vi "MoD Main-Optimize - HPLC Epoxidation Additives Simulation.vi"() -> ()   [LabVIEW 2015]
uses:
  <vilib>/silver_ctls/ArrayMatrixCluster/Real Matrix NI_Silver.ctl
  <vilib>/ni845x/ni845x.llb/ni845xControl.ctl
  <vilib>/addons/control/pid/pid.llb/PID Control Input Filter (DBL).vi
  <vilib>/addons/control/pid/autopid.llb/PID Online Autotuning (Relay Feedback).vi
  <vilib>/Analysis/Matrix/Numeric/Conversions/Array To Matrix - RA2.vi
  <vilib>/addons/control/pid/NI_PID_autopid.lvlib
  <vilib>/addons/control/pid/NI_PID_pid.lvlib
  <vilib>/Analysis/Matrix/NI_Matrix.lvlib
  <vilib>/MakerHub/LINX/LMH-LINX.lvlib
  <vilib>/MakerHub/LINX/Public/Peripherals/Digital/Digital Write 1 Chan.vi
panel:
  out "running?":bool=TRUE
  out "new_reactor_volume":bool[](array[boolean])
  out "new_reactor_length":bool[](array[boolean])
  out "Phase_Sensor_voltage":dbl
  out "P_tot":dbl
  out "pause for ms":bool=TRUE
  out "stop_xl_write":bool=TRUE
  out "Num_exp_till_pause":i32
  out "Syringe_pump?":bool=TRUE
  out "System Error":bool=TRUE
  out "error out":errorcluster
  out "Pump setpoint(ul/min) 6":dbl format="%#_13g"
  out "Pump setpoint(ul/min) 5":dbl format="%#_13g"
  out "Pump setpoint(ul/min) 4":dbl format="%#_13g"
  out "Pump setpoint(ul/min) 3":dbl format="%#_13g"
  out "Pump setpoint(ul/min) 2":dbl format="%#_13g"
  out "Pump setpoint(ul/min) 1":dbl format="%#_13g"
  out "Volume (ul) 5":dbl format="%#_13g"
  out "Volume (ul) 4":dbl format="%#_13g"
  out "Volume (ul) 3":dbl format="%#_13g"
  out "Volume (ul) 2":dbl format="%#_13g"
  out "Volume (ul) 1":dbl format="%#_13g"
  in  "tau 5":dbl format="%#_13g"
  out "tau 4":dbl format="%#_13g"
  out "tau 3":dbl format="%#_13g"
  out "tau 2":dbl format="%#_13g"
  out "tau 1":dbl format="%#_13g"
  out "Reactor Length":dbl format="%#_13g"
  out "Flowrate Sensor 2":dbl format="%#_13g"
  out "Flowrate Sensor 1":dbl format="%#_13g"
  out "Pressure 2":dbl format="%#_13g"
  out "Pressure 1":dbl format="%#_13g"
  out "Temperature Control 5":bool=TRUE
  out "Temperature Control 4":bool=TRUE
  out "Temperature Control 3":bool=TRUE
  out "Temperature Control 2":bool=TRUE
  out "Temperature Control 1":bool=TRUE
  out "Temperature SP 5":dbl format="%#_g'C"
  out "Temperature SP 4":dbl format="%#_g'C"
  out "Temperature SP 3":dbl format="%#_g'C"
  out "Temperature SP 2":dbl format="%#_g'C"
  out "Temperature SP 1":dbl format="%#_g'C"
  in  "Bay Temperature 5":dbl
  in  "SSR Duration 5":dbl
  in  "SSR Duration 4":dbl
  in  "SSR Duration 3":dbl
  in  "SSR Duration 2":dbl
  in  "SSR Duration 1":dbl
  in  "Total Product Amount":dbl=1.0 format="%#_gml"
  out "Setup Error":bool=TRUE
  out "Error Message":string
  out "ID CTR":i32
  in  "Tab Control":T1(tab)
  out "Reagent pic 5":picture
  in  "reagent name 5":string="TFE"
  out "Reagent Pic 4":picture
  in  "reagent name 4":string="ammoniumacetate"
  out "Reagent Pic 3":picture
  in  "reagent  name 3":string="Jacobsen Cat"
  in  "Product name":string="55662-89-0"
  in  "reagent name 1":string="Indene+IS(1M)"
  out "Reagent Pic 1":picture
  in  "Vr5":dbl format="%#_guL"
  in  "Vr4":dbl format="%#_guL"
  in  "Vr3":dbl format="%#_guL"
  in  "Vr2":dbl format="%#_guL"
  in  "Vr1":dbl format="%#_guL"
  in  "System decide help Button":bool
  in  "Reaction Scheme Confirm":bool
  in  "Synthesis Route Array":string[][](array[string])=[["Indene+IS(1M)", "1", "PhB(OH)2", "", "", ""], ["H2O2", "9.76", "-", "-", "-", "-"], ["Jacobsen Cat", "0.025", "-", "-", "-", "-"], ["ammoniumacetate", ".25", "-", "-", "-", "-"], ["TFE", "5", "-", "-", "-", "-"], ["Triflurotoluene", "5", "-", "-", "-", "-"]]
  in  "System decide help Button 2":bool
  out "Setup Confirm":bool=TRUE
  in  "BAY 1":u16(ring) items=["               Bypass", "         Heated Reactor", "    Small Heated Reator", "         Cooled Reactor", "      Packed Bed Reactor", "          Photo Reactor", "             Separator"]
  in  "BAY 5":u16(ring) items=["               Bypass", "         Heated Reactor", "    Small Heated Reactor", "         Cooled Reactor", "     Packed Bed Reactor", "         Photo Reactor", "             Separator"]
  in  "BAY 4":u16(ring) items=["                Bypass", "         Heated Reactor", "    Small Heated Reactor", "         Cooled Reactor", "     Packed Bed Reactor", "         Photo Reactor", "             Separator"]
  in  "BAY 3":u16(ring)=1 items=["               Bypass", "         Heated Reactor", "    Small Heated Reactor", "         Cooled Reactor", "     Packed Bed Reactor", "          Photo Reactor", "             Separator"]
  in  "BAY 2":u16(ring) items=["               Bypass", "         Heated Reactor", "    Small Heated Reactor", "         Cooled Reactor", "      Packed Bed Reactor", "          Photo Reactor", "             Separator"]
  out "Reagent Pic 2":picture
  out "Product Pic":picture
  in  "reagent name 2":string="H2O2"
  in  "reagent name 6":string="Triflurotoluene"
  out "Reagent Pic 6":picture
  in  "System Parameters Help Button":bool
  out "Setup Confirm 2":bool
  in  "System Parameters Confirm Button":bool
  in  "Bay Parameters":T2={"Bay 1 "={"Pump 1 Flowrate"=0.0, "optimize_temp"=FALSE, "optimize_tau"=TRUE, "Run at set flowrate"=FALSE, "Pump 2 Flowrate"=0.0, "Temperature Params"=[40.0, 100.0, 100.0], "pump params 1"=[5.0, 50.0, 325.0], "pump params 2"=[1.0, 10.0, 325.0], "Temperature"=0.0, "Run at set temperature"=FALSE}, "Bay 2 "={"Pump 3 Flowrate"=0.0, "optimize_temp"=FALSE, "optimize_tau"=TRUE, "Run at set flowrate"=FALSE, "Temperature Params"=[40.0, 100.0, 100.0], "Resisdence time params"=[1.0, 15.0, 650.0], "pump_at_ratio"=FALSE, "pump_num_ratio"=4.0, "Temperature"=0.0, "Run at set temperature"=FALSE}, "Bay 3 "={"Pump 4 Flowrate"=100.0, "optimize_temp"=FALSE, "optimize_tau"=TRUE, "Run at set flowrate"=FALSE, "Temperature Params"=[30.0, 50.0, 100.0], "Resisdence time params"=[0.5, 2.0, 0.0], "pump_at_ratio"=FALSE, "pump_num_ratio"=0.05, "Temperature "=0.0, "Run at set temperature"=FALSE}, "Bay 4 "={"Pump 5 Flowrate"=40.0, "Run at set flowrate"=FALSE, "optimize_temp"=FALSE, "optimize_tau"=TRUE, "Resisdence time params"=[0.5, 3.49, 225.0], "Temperature Params"=[40.0, 100.0, 80.0], "pump_at_ratio"=FALSE, "pump_num_ratio"=1.0, "Temperature"=0.0, "Run at set temperature"=FALSE}, "Bay 5 "={"Pump 6 Flowrate"=0.0, "Run at set flowrate"=FALSE, "optimize_temp"=FALSE, "optimize_tau"=FALSE, "Resisdence time params"=[7.62, 114.27, 0.0], "Temperature Params"=[0.0, 0.0, 0.0], "pump_at_ratio"=FALSE, "pump_num_ratio"=0.5, "Temperature"=0.0, "Run at set temperature"=FALSE}, "Excel File Name"="C:\\Users\\HPLC\\Dropbox (MIT)\\MoD Files\\Data\\Epox12182017", "hplc File Name"="C:\\Chem32\\1\\Data\\MOD", "Matlab File"="C:\\Users\\HPLC\\Dropbox (MIT)\\MoD Files\\Data\\Epox12182017", "Syringe for Pump 2?"=TRUE, "Num_conditons_per_wait"=2.0, "Continue from previous optimization?"=FALSE, "Total Number of Experiments 2"=60.0, "Hplc Wait time(min)"=0.25, "increas_decrease_hplc_peak"=FALSE, "Internal Standard?"=TRUE, "ISTD start"=1.2, "ISTD end"=1.9, "hplc_start"=0.7, "hplc_end"=1.1, "throughput_yield"=TRUE} {"Hplc Wait time(min)" format="%#_13g"; "Bay 5"."Temperature Params" format="%#_g'C"; "Bay 4"."Temperature Params" format="%#_g'C"; "Bay 3"."Temperature Params" format="%#_g'C"; "Bay 2"."Temperature Params" format="%#_g'C"; "Bay 1"."Temperature Params" format="%#_g'C"}
  out "System Confirm Not Clicked":string
  out "best_exp_num":dbl=1.0
  out "temperature_best":dbl[](array[numeric])
  out "Flowrates(ul/min)_best":dbl[](array[numeric])
  out "System Status":u16(ring)=2 caption="Sy" items=["System  Error", "System Running", "System Standby"]
  out "Current Experiment":dbl=1.0
  out "Total Number of Experiments":dbl=33.0
  out "Phase Sensor Chart":T3(graph)
  out "HPLC Analysis":bool
  out "Equlibrating Temperature":bool
  out "Flushing System":bool
  out "Calculate condition":bool
  out "Temperature 5":dbl format="%#_g'C"
  out "Temperature 4":dbl format="%#_g'C"
  out "Temperature 3":dbl format="%#_g'C"
  out "Temperature 2":dbl format="%#_g'C"
  out "Temperature 1":dbl format="%#_g'C"
  out "Flowrate Chart":T4(graph)
  out "Teperature Chart":T3(graph)
  out "Pump Setpoints Chart":T3(graph)
  out "Pressure Chart":T3(graph)
  out "Optimization_loop_index":i32
  out "curr_wait_time":dbl
  out "total_flush_time":dbl
  out "Temp SS? 5":bool=TRUE
  out "Temp SS? 4":bool=TRUE
  out "Temp SS? 3":bool=TRUE
  out "Temp SS? 2":bool=TRUE
  out "Temp SS? 1":bool=TRUE
  out "System Flushed?":bool
  out "stop_button clicked":bool
  in  "Pump Addresses":string[](array[string])=["g", "e", "i", "j", "f", "h", ""]
  out "experiment history":T5
  in  "Number of System Flushes per condtion":dbl=2.5
  in  "calculate volume 3":bool=TRUE
  in  "calculate volume 2":bool=TRUE
  in  "calculate volume 1":bool=TRUE
  in  "calculate volume 4":bool
  in  "calculate volume 5":bool
  in  "Extra system dead volume":dbl format="%#_gul"
  in  "new reactor length? 1":bool
  in  "tube_length(in)":dbl[](array[numeric])=[188.0, 188.0, 10.0, 10.0, 10.0]
  out "Pause Before Analysis":bool
  out "Chiller COMM Port":bool
  out "Arduino COMM Port 2":bool
  out "Temperature Sensor COMM Port":bool
  out "Flow Rate":bool
  out "Pressure":bool
  out "Pump COMM Port":bool
  in  "COMM Port :: Milligat Pumps":refnum<visa-resource-name>="COM10"
  in  "Arduino COMM Port":refnum<visa-resource-name>="COM3"
  in  "Sample Valve COMM::Port":refnum<visa-resource-name>="COM4"
  in  "COMM Port:: Harvard Syringe Pump":refnum<visa-resource-name>="COM5"
  in  "tube_id(in)":enum16{".01", ".02", ".03", ".04"}[](array[ring])=[enum.".03", enum.".03", enum.".03", enum.".03", enum.".03"]
  out "Total System Resisdence Time(min)":dbl
  in  "Debug_run_button":bool
  in  "new reactor length? 2":bool
  in  "new reactor length? 3":bool
  in  "new reactor length? 4":bool
  in  "new reactor length? 5":bool
  in  "IR Sensor Device":T6="USB0::0x3923::0x7514::01B3FF21::RAW"
  out "Stop":bool=TRUE
  in  "Run_Stop_cluster":T7
  # "Molecules on Demand"
  # "Synthetic Route"
  # "5"
  # "6"
  # "4"
  # "Product"
  # "1"
  # "2"
  # "3"
  # "Reagent List"
  # "Concentration(M)"
  # "Molecule"
  # "1"
  # "1"
  # "2"
  # "2"
  # "3"
  # "3"
  # "4"
  # "4"
  # "5"
  # "6"
  # "5"
  # "6"
  # "Product"
  # "Reactor Volume:"
  # "Optimization Parameters"
  # "Pause after"
  # "Experiments"
  # "Optimize for"
  # "to"
  # "of HPLC Peak from"
  # "from"
  # "to"
  # "min"
  # "min"
  # "HPLC runtime"
  # "# Iterations"
  # "Reporting"
  # "Excel Output File Name"
  # "HPLC File Path"
  # "MATLAB File Path"
  # "Temperature"
  # "Flowrate(ul/min)"
  # "Lower Bound"
  # "Upper Bound"
  # "Optimize?"
  # "-or-"
  # "Run at"
  # "times incoming flow"
  # "Setpoint"
  # "Temperature"
  # "Flowrate(ul/min)"
  # "Lower Bound"
  # "Upper Bound"
  # "Optimize?"
  # "-or-"
  # "Run at"
  # "times incoming flow"
  # "Setpoint"
  # "Temperature"
  # "Flowrate(ul/min)"
  # "Lower Bound"
  # "Upper Bound"
  # "Optimize?"
  # "-or-"
  # "Run at"
  # "times incoming flow"
  # "Setpoint"
  # "Temperature"
  # "Flowrate 3 (ul/min)"
  # "Lower Bound"
  # "Upper Bound"
  # "Optimize?"
  # "-or-"
  # "Run at"
  # "times incoming flow"
  # "Setpoint"
  # "Temperature"
  # "Flowrate 1(ul/min)"
  # "Flowrate 2(ul/min)"
  # "Lower Bound"
  # "Upper Bound"
  # "Optimize?"
  # "Setpoint"
  # "Pressure (psi)"
  # "System Status"
  # "Temperature('C)"
  # "BAY"
  # "1"
  # "2"
  # "3"
  # "4"
  # "5"
  # "Pump Flowrate Setpoint(ul/min)"
  # "Flowrate (ul/min)"
  # "Phase Sensor"
  # "Current Experiment"
  # "Temperature('C)"
  # "Flowrate(ul/min)"
  # "Exp"
  # "Current Best Condition"
  # "Time to reach steady state:"
  # "Current Wait Time:"
  # "Experimental Steps"
  # "Calculated New Conditions"
  # "Steady State"
  # "Analyzed HPLC"
  # "Equilibrated Temperature"
  # "Tube Length (cm)"
  # "Bay"
  # "Tube ID (in)"
  # "Calculate Volume"
  # "Use new tube length"
  # "1."
  # "2."
  # "3."
  # "4."
  # "5."
  # "Reactor Lengths\n*Heated Reactor - 188cm * Small Reactor - 99cm * Bypass - 10cm * Separator - *"
  # "1"
  # "2"
  # "3"
  # "4"
  # "5"
  # "6"
  # "All Experimental Data"
  # "P1"
  # "P2"
  # "P3"
  # "P4"
  # "P5"
  # "P6"
  # "T1"
  # "T2"
  # "T3"
  # "T4"
  # "T5"
  # "Obj_fun"
  # "HPLC_Data"
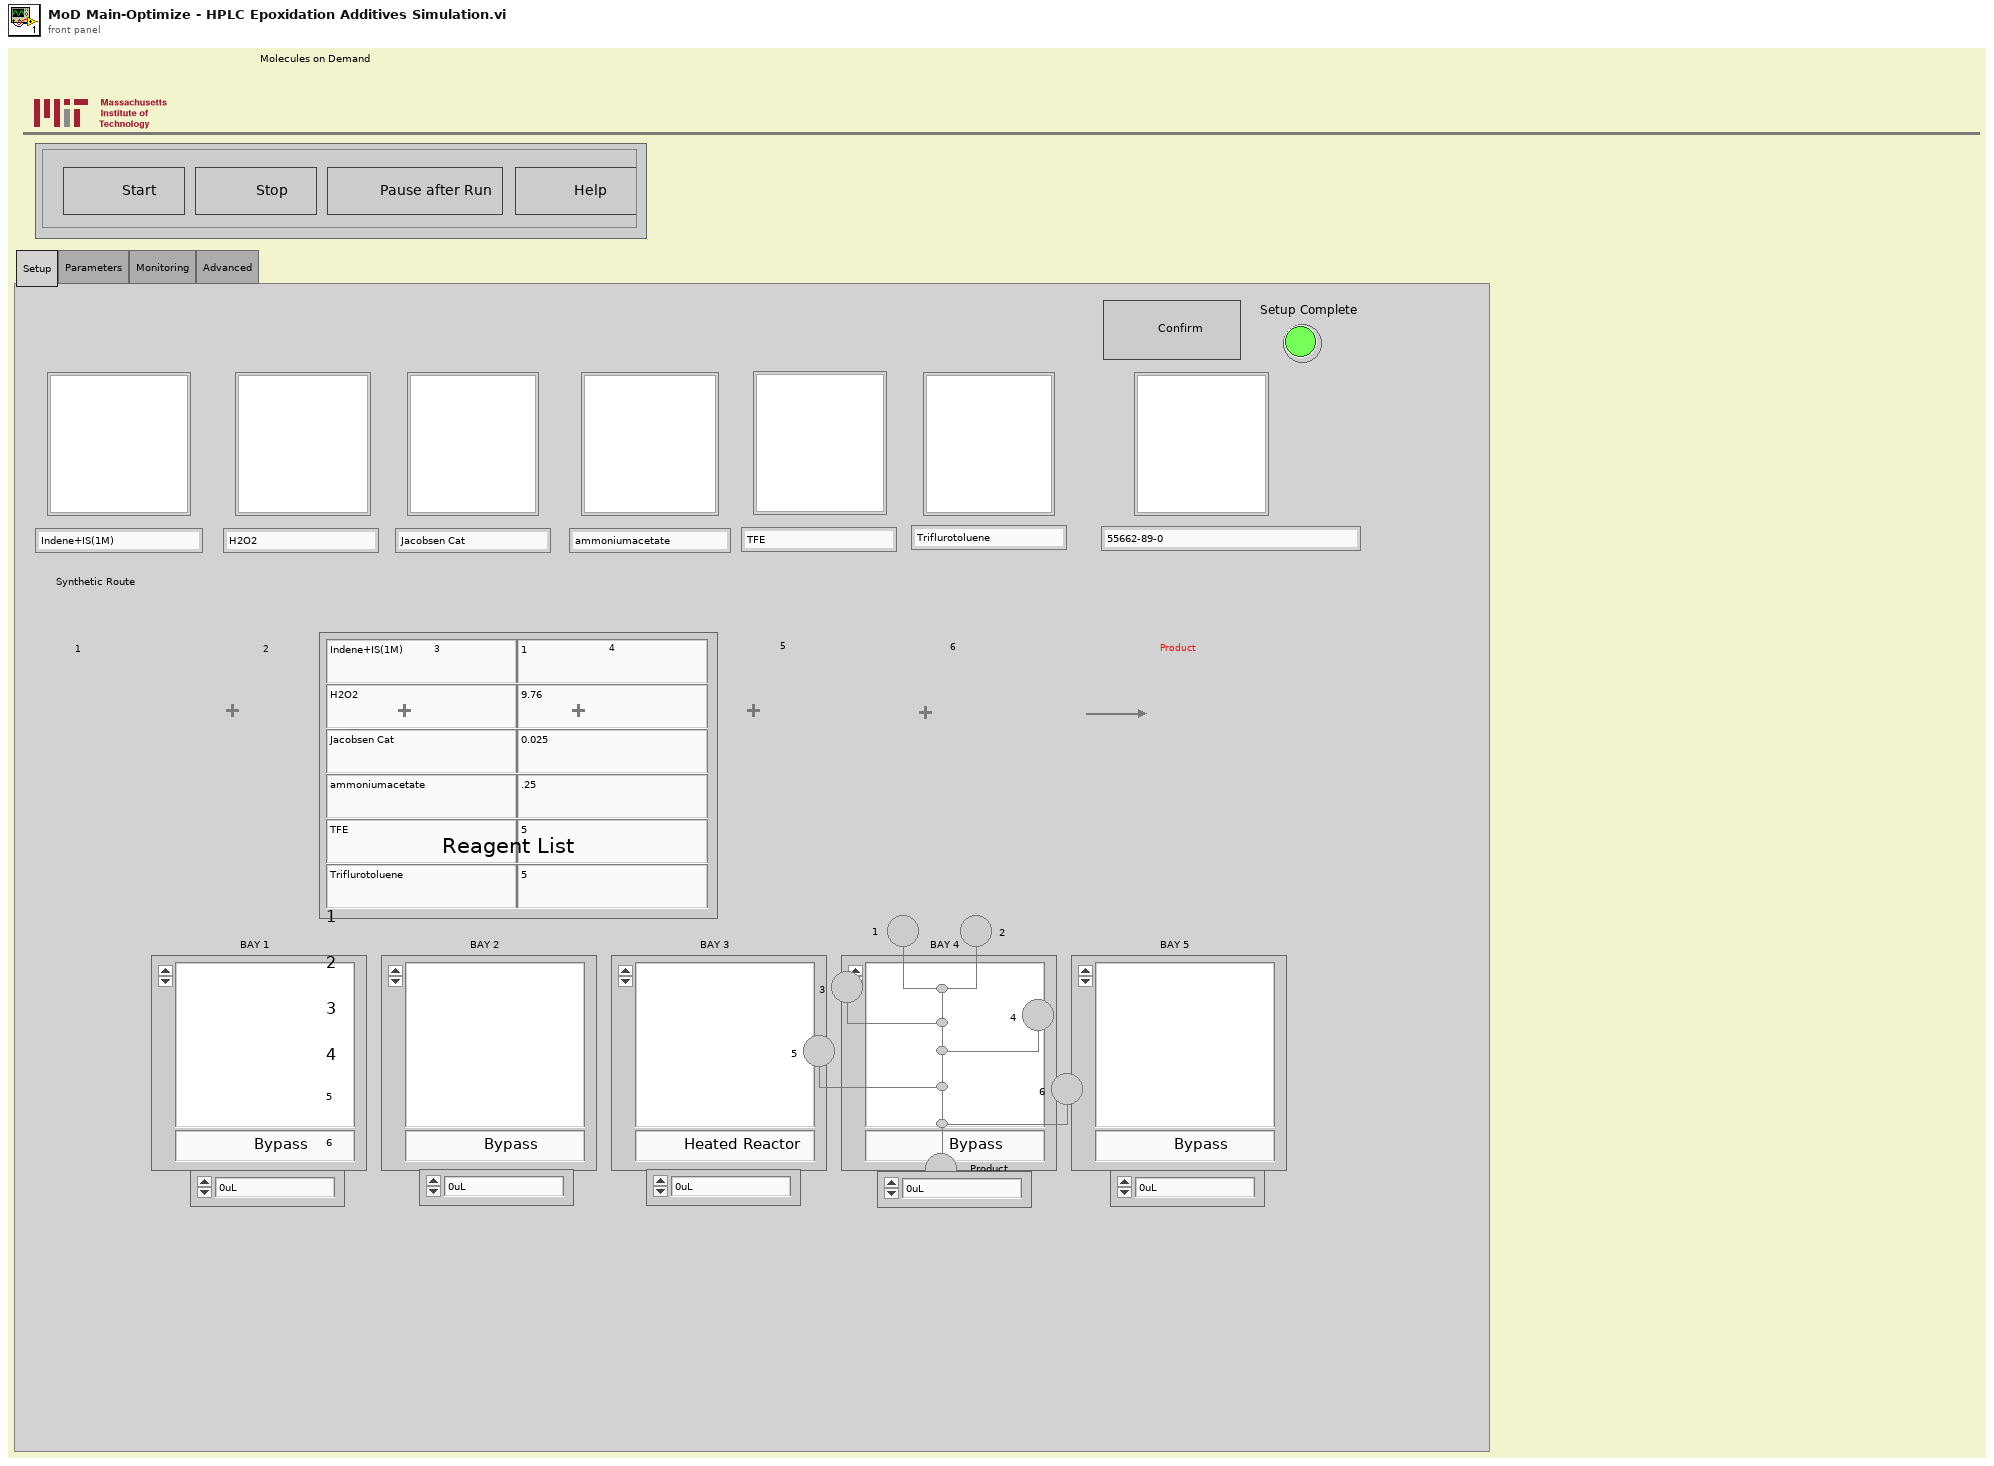
[diagram p1: front panel]
types:
  T1 = enum32{"Setup", "Parameters", "Monitoring", "Advanced"}
  T2 = cluster{"Bay 1 ":cluster{"Pump 1 Flowrate":dbl, "optimize_temp":bool, "optimize_tau":bool, "Run at set flowrate":bool, "Pump 2 Flowrate":dbl, "Temperature Params":dbl[], "pump params 1":dbl[], "pump params 2":dbl[], "Temperature":dbl, "Run at set temperature":bool}, "Bay 2 ":cluster{"Pump 3 Flowrate":dbl, "optimize_temp":bool, "optimize_tau":bool, "Run at set flowrate":bool, "Temperature Params":dbl[], "Resisdence time params":dbl[], "pump_at_ratio":bool, "pump_num_ratio":dbl, "Temperature":dbl, "Run at set temperature":bool}, "Bay 3 ":cluster{"Pump 4 Flowrate":dbl, "optimize_temp":bool, "optimize_tau":bool, "Run at set flowrate":bool, "Temperature Params":dbl[], "Resisdence time params":dbl[], "pump_at_ratio":bool, "pump_num_ratio":dbl, "Temperature ":dbl, "Run at set temperature":bool}, "Bay 4 ":cluster{"Pump 5 Flowrate":dbl, "Run at set flowrate":bool, "optimize_temp":bool, "optimize_tau":bool, "Resisdence time params":dbl[], "Temperature Params":dbl[], "pump_at_ratio":bool, "pump_num_ratio":dbl, "Temperature":dbl, "Run at set temperature":bool}, "Bay 5 ":cluster{"Pump 6 Flowrate":dbl, "Run at set flowrate":bool, "optimize_temp":bool, "optimize_tau":bool, "Resisdence time params":dbl[], "Temperature Params":dbl[], "pump_at_ratio":bool, "pump_num_ratio":dbl, "Temperature":dbl, "Run at set temperature":bool}, "Excel File Name":string, "hplc File Name":string, "Matlab File":string, "Syringe for Pump 2?":bool, "Num_conditons_per_wait":dbl, "Continue from previous optimization?":bool, "Total Number of Experiments 2":dbl, "Hplc Wait time(min)":dbl, "increas_decrease_hplc_peak":bool, "Internal Standard?":bool, "ISTD start":dbl, "ISTD end":dbl, "hplc_start":dbl, "hplc_end":dbl, "throughput_yield":bool}
  T3 = cluster{"[0]":dbl, "[1]":dbl, "[2]":dbl, "[3]":dbl, "[4]":dbl, "[5]":dbl, "[6]":dbl, "[7]":dbl, "[8]":dbl}
  T4 = cluster{"[0]":i32, "[1]":i32, "[2]":i32, "[3]":i32, "[4]":i32, "[5]":i32, "[6]":i32, "[7]":i32, "[8]":i32}
  T5 = typedef "Real Matrix NI_Silver.ctl" = dbl[][]
  T6 = typedef "ni845xControl.ctl" = refnum<k21>
  T7 = cluster{"Stop":bool, "Run":bool, "Stop Run Button":bool, "Help Button":bool}
  T8 = cluster{"Proportional gain Kc":dbl, "Integral time Ti (sec)":dbl, "Derivative time Ti (sec)":dbl}
  T9 = cluster{"type of controller":enum16{"P", "PI", "PID"}, "relay cycles":i32, "relay amplitude":dbl, "control specifications":enum16{"Fast", "Normal", "Slow"}, "PV noise level":dbl}
  T10 = typedef "imagedata.ctl" = cluster{"image type":i32, "image depth":i32, "image":u8[], "mask":u8[], "colors":u32[], "Rectangle":cluster{"left":i16, "top":i16, "right":i16, "bottom":i16}}
  T11 = cluster{"proportional gain (Kc)":dbl, "integral time (Ti, min)":dbl, "derivative time (Td, min)":dbl}
  T12 = typedef "NI_Matrix.lvlib/RealMatrix.ctl" = dbl[][]
  T13 = typedef "LMH-LINX.lvlib/LINX Ref.ctl" = cluster{"IO":T14, "Interface":T15, "LINX Device Config":T16}
  T14 = typedef "LMH-LINX.lvlib/Platform.ctl" = enum16{"Remote", "Local"}
  T15 = typedef "LMH-LINX.lvlib/Interface.ctl" = enum16{"Serial", "TCP"}
  T16 = typedef "LMH-LINX.lvlib/Device.lvlib/LINX Device Config.ctl" = cluster{"Interface":T15, "COM Port":refnum<visa-resource-name>, "TCP Configuration":T17, "Device Family":u8, "Device ID":u8, "Device Name":string, "TCP Ref":refnum<k5>, "Channels":T18}
  T17 = typedef "LMH-LINX.lvlib/Device.lvlib/TCP Config.ctl" = cluster{"IP Address":string, "Port":u16}
  T18 = typedef "LMH-LINX.lvlib/Channels.ctl" = cluster{"DI":u8[], "DO":u8[], "AI":u8[], "AO":u8[], "PWM":u8[], "QE":u8[], "UART":u8[], "I2C 2":u8[], "SPI":u8[], "CAN":u8[], "Servo":u8[], "AI Ref (V)":dbl, "AI Resolution (Bits)":u8, "AO Ref (V)":dbl, "AO Resolution (Bits)":u8}
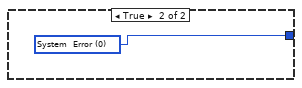
[diagram p4: hidden frame]
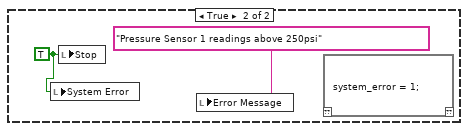
[diagram p6: hidden frame]
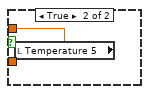
[diagram p7: hidden frame]
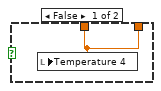
[diagram p8: hidden frame]
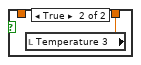
[diagram p9: hidden frame]
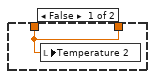
[diagram p10: hidden frame]
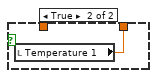
[diagram p11: hidden frame]
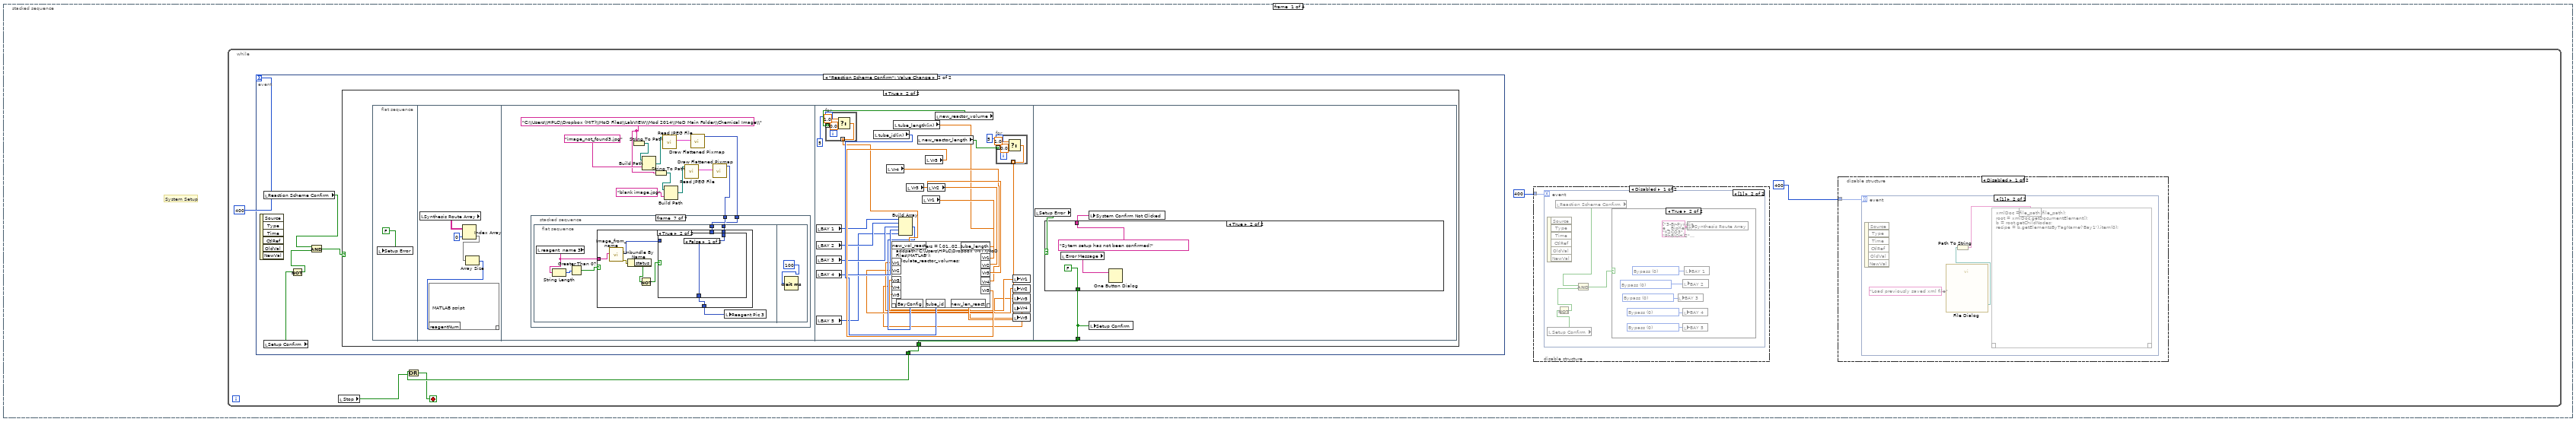
[diagram p12: hidden frame]
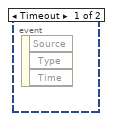
[diagram p13: hidden frame]
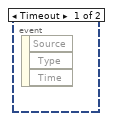
[diagram p15: hidden frame]
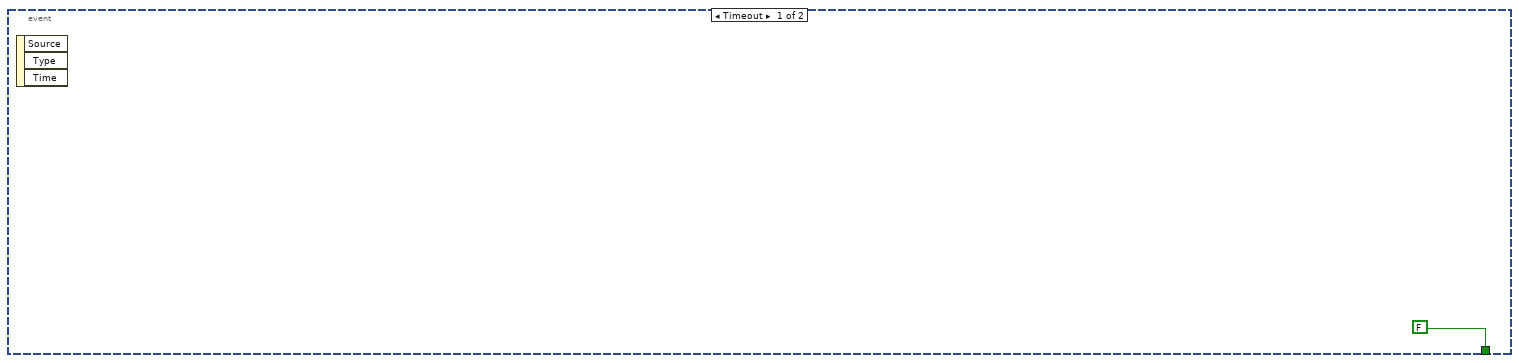
[diagram p18: hidden frame]
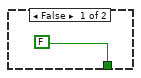
[diagram p19: hidden frame]
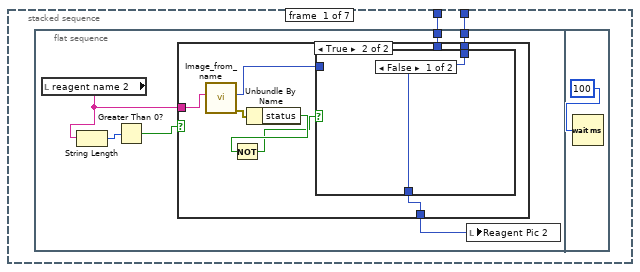
[diagram p20: hidden frame]
diagram:
  # "Assume User always uses the first bay first"
  n1 = flat-sequence {
    tunnel: ["COMM Port :: Milligat Pumps"] -> w4
    tunnel: ["Arduino COMM Port"] -> w3
    tunnel: ["Bay Parameters"] -> w1
    tunnel: [w50] -> w5
    tunnel: w4 -> [w50]
    tunnel: w3 -> [_]
    tunnel: [w44] -> w2
    tunnel: w1 -> [w41]
    tunnel: w5 -> [w54]
    tunnel: w2 -> [w53]
    frame #0 {
      w29 = FALSE ("Equlibrating Temperature")
      n2 = script code="TempArr1=[23 23 23 23 23 23 23 23 23 23]';\nTempArr2=[23 23 23 23 23 23 23 23 23 23]';\nTempArr3=[23 23 23 23 23 23 23 23 23 23]';\nTempArr4=[23 23 23 23 23 23 23 23 23 23]';\nTempArr5=[23 23 23 23 23 23 23 23 23 23]';\nTempArrLED=[23 23 23 23 23 23 23 23 23 23]';\ntemp_error1 =0;\ntemp_error2 =0;\ntemp_error3 =0;\ntemp_error4 =0;\ntemp_error5 =0;\ntemp_check1 = 0;\ntemp_check2 = 0;\ntemp_check3 = 0;\ntemp_check4 = 0;\ntemp_check5 = 0;\nT1=23;\nT2=23;\nT3=23;\nT4=23;\nT5=23;"() -> ()  [unwired: 1 in, 1 out]
      n3 = Build Array("calculate volume 1", "calculate volume 2", "calculate volume 3", "calculate volume 4", "calculate volume 5") -> (→"new_reactor_volume":bool[])
      n4 = Build Array("new reactor length? 1", "new reactor length? 2", "new reactor length? 3", "new reactor length? 4", "new reactor length? 5") -> (→"new_reactor_length":bool[])
      "Stop" <- FALSE ("Stop")
      "ID CTR" <- 0
      "Setup Confirm" <- FALSE ("Setup Confirm")
      "Error Message" <- "System shutdown sucessfully. No errors to report." ("Error Message")
      "Setup Error" <- FALSE ("Setup Error")
      "Reactor Length" <- 10.5
      "System Error" <- FALSE ("System Error")
      "Num_exp_till_pause" <- 0 ("Num_exp_till_pause")
      "Equlibrating Temperature" <- w29
      "Calculate condition" <- w29
      "Flushing System" <- w29
      "HPLC Analysis" <- w29
      "stop_xl_write" <- FALSE ("stop_xl_write")
      "Pump setpoint(ul/min) 1" <- 0.0 ("Pump setpoint(ul/min) 1")
      "Pump setpoint(ul/min) 2" <- 0.0 ("Pump setpoint(ul/min) 2")
      "Pump setpoint(ul/min) 4" <- 0.0 ("Pump setpoint(ul/min) 4")
      "Pump setpoint(ul/min) 6" <- 0.0 ("Pump setpoint(ul/min) 6")
      "Pump setpoint(ul/min) 3" <- 0.0 ("Pump setpoint(ul/min) 3")
      "Pump setpoint(ul/min) 5" <- 0.0 ("Pump setpoint(ul/min) 5")
      "pause for ms" <- FALSE ("pause for ms")
      "Setup Confirm 2" <- FALSE ("Setup Confirm 2")
      "running?" <- FALSE ("running?")
    }
    frame #1 {
      w40 = FALSE
      w49 = 23
      (unwired) path "C:/Users/User1/Documents/Lab/MoD/Images"
      n5 = disable-structure shown="Disabled" {
        frame Disabled {
          n6 = local read "BAY 2"() -> ()  [unwired: 1 out]
          n7 = local read "BAY 3"() -> ()  [unwired: 1 out]
          n8 = local read "BAY 4"() -> ()  [unwired: 1 out]
          n9 = local read "BAY 5"() -> ()  [unwired: 1 out]
          n10 = local read "BAY 1"() -> ()  [unwired: 1 out]
        }
        frame Enabled {
        }
      }
      n11 = local write "Debug_run_button"(TRUE) -> ()
      n12 = local write "System Parameters Confirm Button"(w40) -> ()
      n13 = local write "Setup Confirm 2"(w40) -> ()
      n14 = Unbundle By Name(w41) -> ("Syringe for Pump 2?"=→"Syringe_pump?":bool)
      n15 = local write "Temperature 1"(w49) -> ()
      n16 = local write "Temperature 2"(w49) -> ()
      n17 = local write "Temperature 3"(w49) -> ()
      n18 = local write "Temperature 4"(w49) -> ()
      n19 = local write "Temperature 5"(w49) -> ()
      n20 = local write "Temperature SP 1"(w49) -> ()
      n21 = local write "Temperature SP 2"(w49) -> ()
      n22 = local write "Temperature SP 3"(w49) -> ()
      n23 = local write "Temperature SP 4"(w49) -> ()
      n24 = local write "Temperature SP 5"(w49) -> ()
      n25 = Current VI's Path() -> (path=w48:path)
      n26 = Strip Path(path=w48) -> (stripped path=w46:path)  [unwired: 1 out]
      n27 = Strip Path(path=w46) -> (stripped path=w45:path)  [unwired: 1 out]
      n28 = Build Path(base path=w45, name or relative path="MATLAB") -> (appended path=w44:path)
    }
    frame #2 {
      # "Main Help Dialog Popup"
      n29 = while {
        stop <- w1206 stop-if-true
        n30 = event shown="[6] \"Run_Stop_cluster.Run\": Value Change" {
          selector: _ -> [_ _ _ _ _ _ _]
          dyn-events: _ -> [_ _ _ _ _ _ _]
          timeout: 100 -> [_ _ _ _ _ _ _]
          event Timeout {
            n31 = event-data() -> ()  [unwired: 1 in, 3 out]
          }
          event "Run_Stop_cluster.Help Button": Value Change {
            n32 = local read "Run_Stop_cluster"() -> (w1209:T7)
            n33 = event-data() -> ()  [unwired: 1 in, 4 out]
            n34 = Unbundle By Name(w1209) -> ("Help Button"=w1208:bool)
            n35 = case shown="True" w1208 {
              frame False {
              }
              frame True {
                n36 = call "help.vi"() -> ()  [unwired: 11 in]
              }
            }
          }
          event "System decide help Button": Value Change {
            n37 = event-data() -> ()  [unwired: 1 in, 5 out]
            n38 = call "help_synthesis_man-auto_instructions.vi"() -> ()  [unwired: 12 in]
          }
          event "System Parameters Help Button": Value Change {
            n39 = event-data() -> ()  [unwired: 1 in, 5 out]
            n40 = call "help_parameters_setup.vi"() -> ()  [unwired: 12 in]
          }
          event "System decide help Button 2": Value Change {
            n41 = event-data() -> ()  [unwired: 1 in, 5 out]
            n42 = call "help_synthesis_route_instructions.vi"() -> ()  [unwired: 12 in]
          }
          event "Run_Stop_cluster.Stop": Value Change {
            n43 = event-data() -> ()  [unwired: 1 in, 5 out]
            n44 = local write "Stop"(TRUE) -> ()
          }
          event "Run_Stop_cluster.Run": Value Change {
            n45 = event-data() -> ()  [unwired: 1 in, 5 out]
            n46 = local write "running?"(TRUE) -> ()
          }
        }
        n47 = local read "Stop"() -> (w1206:bool)
      }
      n48 = stacked-sequence {
        tunnel: w54 -> [_ _ _ _]
        tunnel: w53 -> [_ w392 _ _]
        frame #0 {
          # "System Setup"
          n49 = while {
            stop <- w167 stop-if-true
            n50 = event shown="[1] \"Reaction Scheme Confirm\": Value Change" {
              selector: _ -> [_ _]
              dyn-events: _ -> [_ _]
              timeout: 400 -> [_ _]
              tunnel: [FALSE w187] -> w169
              event Timeout {
                n51 = event-data() -> ()  [unwired: 1 in, 3 out]
              }
              event "Reaction Scheme Confirm": Value Change {
                n52 = event-data() -> ()  [unwired: 1 in, 6 out]
                n53 = local read "Reaction Scheme Confirm"() -> (w191:bool)
                n54 = local read "Setup Confirm"() -> (w189:bool)
                n55 = Not(x=w189) -> (.not. x?=w188:bool)
                n56 = And(x=w191, y=w188) -> (x .and. y?=w190:bool)
                n57 = case shown="True" w190 {
                  tunnel: [FALSE w193] -> w187
                  frame False {
                  }
                  frame True {
                    n58 = flat-sequence {
                      tunnel: [w382] -> w193
                      frame #0 {
                        n59 = local write "Setup Error"(FALSE) -> ()
                      }
                      frame #1 {
                        n60 = local read "Synthesis Route Array"() -> (w197:string[][])
                        n61 = Index Array(array=w197, index (col)=0 ("disabled index (col)")) -> (element=w195:string[])  [unwired: 1 in]
                        n62 = Array Size(array=w195) -> (size(s)=w198:i32)
                        n63 = script code="MATLAB script"("reagentNum"=w198) -> ()  [unwired: 1 in, 1 out]
                      }
                      frame #2 {
                        w201 = "C:\\Users\\HPLC\\Dropbox (MIT)\\MoD Files\\LabVIEW\\Mod 2014\\MoD Main Folder\\Chemical Image\\" ("string")
                        n64 = String To Path(string=w201) -> (path=w207:path)
                        n65 = Build Path(base path=w207, name or relative path="image_not_found3.jpg") -> (appended path=w206:path)
                        n66 = String To Path(string=w201) -> (path=w204:path)
                        n67 = call <vilib>:"Read JPEG File.vi"("path to JPEG file"=w206) -> ("image data"=w209:T10)  [unwired: 1 in, 9 out]
                        n68 = Build Path(base path=w204, name or relative path="blank image.jpg") -> (appended path=w202:path)
                        n69 = call <vilib>:"Read JPEG File.vi"("path to JPEG file"=w202) -> ("image data"=w205:T10)  [unwired: 1 in, 9 out]
                        n70 = call <vilib>:"Draw Flattened Pixmap.vi"("image data"=w209) -> ("new picture"=w200:picture)  [unwired: 3 in, 5 out]
                        n71 = call <vilib>:"Draw Flattened Pixmap.vi"("image data"=w205) -> ("new picture"=w199:picture)  [unwired: 3 in, 5 out]
                        n72 = stacked-sequence {
                          tunnel: w200 -> [w211 w231 w251 w271 w291 w310 w330]
                          tunnel: w199 -> [w210 w230 w250 w270 w290 w311 w331]
                          frame #0 {
                            n73 = flat-sequence {
                              tunnel: w211 -> [w217]
                              tunnel: w210 -> [w215]
                              frame #0 {
                                n74 = local read "reagent name 2"() -> (w213:string)
                                n75 = String Length(string=w213) -> (length=w216:i32)
                                n76 = Greater Than 0?(x=w216) -> (x > 0?=w214:bool)
                                n77 = case shown="True" w214 {
                                tunnel: w217 -> [_ w223]
                                tunnel: w215 -> [w218 _]
                                tunnel: [w218 w222] -> w212
                                tunnel: w213 -> [_ w221]
                                frame False {
                                }
                                frame True {
                                n78 = call "Image_from_name.vi"("Chemical Name"=w221) -> ("error out"=w224:errorcluster, "Downloaded Picture"=w225:picture)  [unwired: 8 in, 1 out]
                                n79 = Unbundle By Name(w224) -> ("status"=w220:bool)
                                n80 = Not(x=w220) -> (.not. x?=w219:bool)
                                n81 = case shown="False" w219 {
                                tunnel: w225 -> [_ w228]
                                tunnel: [w226 w227] -> w222
                                tunnel: w223 -> [w226 _]
                                frame False {
                                }
                                frame True {
                                n82 = call <vilib>:"Draw Flattened Pixmap.vi"("picture"=w228) -> ("new picture"=w227:picture)  [unwired: 8 in]
                                }
                                }
                                }
                                }
                                n83 = local write "Reagent Pic 2"(w212) -> ()
                              }
                              frame #1 {
                                n84 = Wait (ms)(milliseconds to wait=100) -> ()  [unwired: 1 out]
                              }
                            }
                          }
                          frame #1 {
                            n85 = flat-sequence {
                              tunnel: w231 -> [w237]
                              tunnel: w230 -> [w235]
                              frame #0 {
                                n86 = local read "reagent name 1"() -> (w232:string)
                                n87 = String Length(string=w232) -> (length=w236:i32)
                                n88 = Greater Than 0?(x=w236) -> (x > 0?=w234:bool)
                                n89 = case shown="True" w234 {
                                tunnel: w237 -> [_ w243]
                                tunnel: w235 -> [w238 _]
                                tunnel: [w238 w242] -> w233
                                tunnel: w232 -> [_ w241]
                                frame False {
                                }
                                frame True {
                                n90 = call "Image_from_name.vi"("Chemical Name"=w241) -> ("error out"=w244:errorcluster, "Downloaded Picture"=w245:picture)  [unwired: 8 in, 1 out]
                                n91 = Unbundle By Name(w244) -> ("status"=w240:bool)
                                n92 = Not(x=w240) -> (.not. x?=w239:bool)
                                n93 = case shown="True" w239 {
                                tunnel: w245 -> [_ w248]
                                tunnel: [w246 w247] -> w242
                                tunnel: w243 -> [w246 _]
                                frame False {
                                }
                                frame True {
                                n94 = call <vilib>:"Draw Flattened Pixmap.vi"("picture"=w248) -> ("new picture"=w247:picture)  [unwired: 8 in]
                                }
                                }
                                }
                                }
                                n95 = local write "Reagent Pic 1"(w233) -> ()
                              }
                              frame #1 {
                                n96 = Wait (ms)(milliseconds to wait=100) -> ()  [unwired: 1 out]
                              }
                            }
                          }
                          frame #2 {
                            n97 = flat-sequence {
                              tunnel: w251 -> [w257]
                              tunnel: w250 -> [w255]
                              frame #0 {
                                n98 = local read "Product name"() -> (w252:string)
                                n99 = String Length(string=w252) -> (length=w256:i32)
                                n100 = Greater Than 0?(x=w256) -> (x > 0?=w254:bool)
                                n101 = case shown="True" w254 {
                                tunnel: w257 -> [_ w263]
                                tunnel: w255 -> [w258 _]
                                tunnel: [w258 w262] -> w253
                                tunnel: w252 -> [_ w261]
                                frame False {
                                }
                                frame True {
                                n102 = call "Image_from_name.vi"("Chemical Name"=w261) -> ("error out"=w264:errorcluster, "Downloaded Picture"=w265:picture)  [unwired: 8 in, 1 out]
                                n103 = Unbundle By Name(w264) -> ("status"=w259:bool)
                                n104 = Not(x=w259) -> (.not. x?=w260:bool)
                                n105 = case shown="False" w260 {
                                tunnel: w265 -> [_ w268]
                                tunnel: [w266 w267] -> w262
                                tunnel: w263 -> [w266 _]
                                frame False {
                                }
                                frame True {
                                n106 = call <vilib>:"Draw Flattened Pixmap.vi"("picture"=w268) -> ("new picture"=w267:picture)  [unwired: 8 in]
                                }
                                }
                                }
                                }
                                n107 = local write "Product Pic"(w253) -> ()
                              }
                              frame #1 {
                                n108 = Wait (ms)(milliseconds to wait=100) -> ()  [unwired: 1 out]
                              }
                            }
                          }
                          frame #3 {
                            n109 = flat-sequence {
                              tunnel: w271 -> [w277]
                              tunnel: w270 -> [w275]
                              frame #0 {
                                n110 = local read "reagent name 6"() -> (w272:string)
                                n111 = String Length(string=w272) -> (length=w276:i32)
                                n112 = Greater Than 0?(x=w276) -> (x > 0?=w274:bool)
                                n113 = case shown="True" w274 {
                                tunnel: w277 -> [_ w283]
                                tunnel: w275 -> [w278 _]
                                tunnel: [w278 w282] -> w273
                                tunnel: w272 -> [_ w281]
                                frame False {
                                }
                                frame True {
                                n114 = call "Image_from_name.vi"("Chemical Name"=w281) -> ("error out"=w284:errorcluster, "Downloaded Picture"=w285:picture)  [unwired: 8 in, 1 out]
                                n115 = Unbundle By Name(w284) -> ("status"=w279:bool)
                                n116 = Not(x=w279) -> (.not. x?=w280:bool)
                                n117 = case shown="False" w280 {
                                tunnel: w285 -> [_ w288]
                                tunnel: [w286 w287] -> w282
                                tunnel: w283 -> [w286 _]
                                frame False {
                                }
                                frame True {
                                n118 = call <vilib>:"Draw Flattened Pixmap.vi"("picture"=w288) -> ("new picture"=w287:picture)  [unwired: 8 in]
                                }
                                }
                                }
                                }
                                n119 = local write "Reagent Pic 6"(w273) -> ()
                              }
                              frame #1 {
                                n120 = Wait (ms)(milliseconds to wait=100) -> ()  [unwired: 1 out]
                              }
                            }
                          }
                          frame #4 {
                            n121 = flat-sequence {
                              tunnel: w291 -> [w297]
                              tunnel: w290 -> [w295]
                              frame #0 {
                                n122 = local read "reagent name 5"() -> (w292:string)
                                n123 = String Length(string=w292) -> (length=w296:i32)
                                n124 = Greater Than 0?(x=w296) -> (x > 0?=w294:bool)
                                n125 = case shown="True" w294 {
                                tunnel: w297 -> [_ w303]
                                tunnel: w295 -> [w298 _]
                                tunnel: [w298 w302] -> w293
                                tunnel: w292 -> [_ w301]
                                frame False {
                                }
                                frame True {
                                n126 = call "Image_from_name.vi"("Chemical Name"=w301) -> ("error out"=w304:errorcluster, "Downloaded Picture"=w305:picture)  [unwired: 8 in, 1 out]
                                n127 = Unbundle By Name(w304) -> ("status"=w299:bool)
                                n128 = Not(x=w299) -> (.not. x?=w300:bool)
                                n129 = case shown="False" w300 {
                                tunnel: w305 -> [_ w308]
                                tunnel: [w306 w307] -> w302
                                tunnel: w303 -> [w306 _]
                                frame False {
                                }
                                frame True {
                                n130 = call <vilib>:"Draw Flattened Pixmap.vi"("picture"=w308) -> ("new picture"=w307:picture)  [unwired: 8 in]
                                }
                                }
                                }
                                }
                                n131 = local write "Reagent pic 5"(w293) -> ()
                              }
                              frame #1 {
                                n132 = Wait (ms)(milliseconds to wait=100) -> ()  [unwired: 1 out]
                              }
                            }
                          }
                          frame #5 {
                            n133 = flat-sequence {
                              tunnel: w311 -> [w315]
                              tunnel: w310 -> [w314]
                              frame #0 {
                                n134 = local read "reagent name 4"() -> (w312:string)
                                n135 = String Length(string=w312) -> (length=w317:i32)
                                n136 = Greater Than 0?(x=w317) -> (x > 0?=w316:bool)
                                n137 = case shown="True" w316 {
                                tunnel: w314 -> [_ w323]
                                tunnel: w315 -> [w318 _]
                                tunnel: [w318 w322] -> w313
                                tunnel: w312 -> [_ w321]
                                frame False {
                                }
                                frame True {
                                n138 = call "Image_from_name.vi"("Chemical Name"=w321) -> ("error out"=w324:errorcluster, "Downloaded Picture"=w325:picture)  [unwired: 8 in, 1 out]
                                n139 = Unbundle By Name(w324) -> ("status"=w319:bool)
                                n140 = Not(x=w319) -> (.not. x?=w320:bool)
                                n141 = case shown="False" w320 {
                                tunnel: w325 -> [_ w328]
                                tunnel: [w326 w327] -> w322
                                tunnel: w323 -> [w326 _]
                                frame False {
                                }
                                frame True {
                                n142 = call <vilib>:"Draw Flattened Pixmap.vi"("picture"=w328) -> ("new picture"=w327:picture)  [unwired: 8 in]
                                }
                                }
                                }
                                }
                                n143 = local write "Reagent Pic 4"(w313) -> ()
                              }
                              frame #1 {
                                n144 = Wait (ms)(milliseconds to wait=100) -> ()  [unwired: 1 out]
                              }
                            }
                          }
                          frame #6 {
                            n145 = flat-sequence {
                              tunnel: w331 -> [w335]
                              tunnel: w330 -> [w334]
                              frame #0 {
                                n146 = local read "reagent  name 3"() -> (w332:string)
                                n147 = String Length(string=w332) -> (length=w337:i32)
                                n148 = Greater Than 0?(x=w337) -> (x > 0?=w336:bool)
                                n149 = case shown="True" w336 {
                                tunnel: w334 -> [_ w343]
                                tunnel: w335 -> [w338 _]
                                tunnel: [w338 w342] -> w333
                                tunnel: w332 -> [_ w341]
                                frame False {
                                }
                                frame True {
                                n150 = call "Image_from_name.vi"("Chemical Name"=w341) -> ("error out"=w344:errorcluster, "Downloaded Picture"=w345:picture)  [unwired: 8 in, 1 out]
                                n151 = Unbundle By Name(w344) -> ("status"=w339:bool)
                                n152 = Not(x=w339) -> (.not. x?=w340:bool)
                                n153 = case shown="False" w340 {
                                tunnel: w345 -> [_ w348]
                                tunnel: [w346 w347] -> w342
                                tunnel: w343 -> [w346 _]
                                frame False {
                                }
                                frame True {
                                n154 = call <vilib>:"Draw Flattened Pixmap.vi"("picture"=w348) -> ("new picture"=w347:picture)  [unwired: 8 in]
                                }
                                }
                                }
                                }
                                n155 = local write "Reagent Pic 3"(w333) -> ()
                              }
                              frame #1 {
                                n156 = Wait (ms)(milliseconds to wait=100) -> ()  [unwired: 1 out]
                              }
                            }
                          }
                        }
                      }
                      frame #3 {
                        n157 = local read "BAY 1"() -> (w360:u16)
                        n158 = local read "BAY 2"() -> (w359:u16)
                        n159 = local read "BAY 3"() -> (w358:u16)
                        n160 = local read "BAY 4"() -> (w357:u16)
                        n161 = local read "BAY 5"() -> (w356:u16)
                        n162 = local read "tube_id(in)"() -> (w367:enum16{".01", ".02", ".03", ".04"}[])
                        n163 = local read "Vr4"() -> (w370:dbl)
                        n164 = local read "tube_length(in)"() -> (w368:dbl[])
                        n165 = Build Array(w360, w359, w358, w357, w356) -> (w355:u16[])
                        n166 = local read "Vr3"() -> (w371:dbl)
                        n167 = local read "new_reactor_length"() -> (w365:bool[])
                        n168 = local read "Vr1"() -> (w373:dbl)
                        n169 = local read "Vr5"() -> (w369:dbl)
                        n170 = local read "Vr2"() -> (w372:dbl)
                        n171 = local read "new_reactor_volume"() -> (w363:bool[])
                        n172 = for {
                          N: 5 -> [_]
                          tunnel: w363 -> [w377] mode=indexing
                          tunnel: [w374] -> w361 mode=indexing
                          n173 = Select(t=1.0, s=w377, f=0.0) -> (s? t:f=w374:dbl)
                        }
                        n174 = for {
                          N: 5 -> [_]
                          tunnel: w365 -> [w381] mode=indexing
                          tunnel: [w378] -> w364 mode=indexing
                          n175 = Select(t=1.0, s=w381, f=0.0) -> (s? t:f=w378:dbl)
                        }
                        n176 = script code="tube_diameters = [.01,.02,.03,.04];\naddpath('C:\\Users\\HPLC\\Dropbox (MIT)\\MoD Files\\MATLAB');\ncalculate_reactor_volumes;"("BayConfig"=w355, "Vr1"=w373, "Vr2"=w372, "Vr3"=w371, "Vr4"=w370, "Vr5"=w369, "tube_length"=w368, "tube_id"=w367, "new_len_react"=w364, "new_vol_react"=w361) -> ("Vr1"=w354:dbl, "Vr2"=w353:dbl, "Vr3"=w352:dbl, "Vr4"=w351:dbl, "Vr5"=w350:dbl)  [unwired: 1 in, 1 out]
                        n177 = local write "Vr1"(w354) -> ()
                        n178 = local write "Vr2"(w353) -> ()
                        n179 = local write "Vr3"(w352) -> ()
                        n180 = local write "Vr4"(w351) -> ()
                        n181 = local write "Vr5"(w350) -> ()
                      }
                      frame #4 {
                        n182 = local read "Setup Error"() -> (w384:bool)
                        n183 = case shown="True" w384 {
                          tunnel: [TRUE FALSE] -> w382
                          tunnel: ["" "Sytem setup has not been confirmed!"] -> w383
                          frame False {
                          }
                          frame True {
                            n184 = local read "Error Message"() -> (w389:string)
                            n185 = One Button Dialog(message=w389) -> ()  [unwired: 1 in, 1 out]
                          }
                        }
                        n186 = local write "System Confirm Not Clicked"(w383) -> ()
                        n187 = local write "Setup Confirm"(w382) -> ()
                      }
                    }
                  }
                }
              }
            }
            n188 = local read "Stop"() -> (w168:bool)
            n189 = Or(x=w169, y=w168) -> (x .or. y?=w167:bool)
            n190 = disable-structure shown="Disabled" {
              disable-tunnel: 400 -> [w175 _]
              frame Disabled {
                n191 = event shown="[1]" {
                  selector: _ -> [_ _]
                  dyn-events: _ -> [_ _]
                  timeout: w175 -> [_ _]
                  event Timeout {
                    n192 = event-data() -> ()  [unwired: 1 in, 3 out]
                  }
                  event #1 (no event record) {
                    n193 = event-data() -> ()  [unwired: 1 in, 6 out]
                    n194 = local read "Setup Confirm"() -> (w176:bool)
                    n195 = local read "Reaction Scheme Confirm"() -> (w177:bool)
                    n196 = Not(x=w176) -> (.not. x?=w179:bool)
                    n197 = And(x=w177, y=w179) -> (x .and. y?=w178:bool)
                    n198 = case shown="True" w178 {
                      frame False {
                      }
                      frame True {
                        w181 = u16 0 items=["                     Bypass", "                Hot Reactor", "                 Separator"] ("BAY 5")
                        w182 = u16 0 items=["                     Bypass", "                Hot Reactor", "                  Separator"] ("BAY 4")
                        w183 = u16 0 items=["                     Bypass", "                 Hot Reactor", "                  Separator"] ("BAY 3")
                        w184 = u16 0 items=["                     Bypass", "                Hot Reactor", "                  Separator"] ("BAY 2")
                        w185 = u16 0 items=["                 Bypass", "             Hot Reactor", "               Separator"] ("BAY 1")
                        n199 = local write "BAY 3"(w183) -> ()
                        n200 = local write "BAY 4"(w182) -> ()
                        n201 = local write "BAY 5"(w181) -> ()
                        n202 = local write "BAY 2"(w184) -> ()
                        n203 = local write "BAY 1"(w185) -> ()
                        n204 = local write "Synthesis Route Array"(string[][] [["3-Br-Pyridine _ Biphenyl", "K2CO3", "PhB(OH)2", "", "", ""]] ("Synthesis Route Array")) -> ()
                      }
                    }
                  }
                }
              }
              frame Enabled {
              }
            }
            n205 = disable-structure shown="Disabled" {
              disable-tunnel: 400 -> [w171 _]
              frame Disabled {
                n206 = event shown="[1]" {
                  selector: _ -> [_ _]
                  dyn-events: _ -> [_ _]
                  timeout: w171 -> [_ _]
                  event Timeout {
                    n207 = event-data() -> ()  [unwired: 1 in, 3 out]
                  }
                  event #1 (no event record) {
                    n208 = event-data() -> ()  [unwired: 1 in, 6 out]
                    n209 = call "File Dialog"("prompt"="Load previously saved xml file") -> ("selected path"=w173:path)  [unwired: 11 in, 3 out]
                    n210 = Path To String(path=w173) -> (string=w172:string)
                    n211 = script code="xmlDoc = xmlread(file_path);\nroot = xmlDoc.getDocumentElement();\nb = root.getChildNodes;\nrecipe = b.getElementsByTagName('Bay1').item(0);"("file_path"=w172) -> ()  [unwired: 1 in, 1 out]
                  }
                }
              }
              frame Enabled {
              }
            }
          }
        }
        frame #1 {
          n212 = local read "Stop"() -> (w391:bool)
          n213 = Not(x=w391) -> (.not. x?=w390:bool)
          n214 = case shown="True" w390 {
            tunnel: w392 -> [_ w395]
            frame False {
              "stop_button clicked" <- TRUE ("stop_button clicked")
            }
            frame True {
              # "Parameters Initilization"
              n215 = flat-sequence {
                tunnel: w395 -> [w397]
                tunnel: [w396] -> w394
                tunnel: w394 -> [w556]
                frame #0 {
                  # "Setup bays(RFID - verify)"
                  n216 = disable-structure shown="Disabled" {
                    frame Disabled {
                      n217 = local read "BAY 1"() -> ()  [unwired: 1 out]
                      n218 = local read "BAY 2"() -> ()  [unwired: 1 out]
                      n219 = local read "BAY 3"() -> ()  [unwired: 1 out]
                      n220 = local read "BAY 4"() -> ()  [unwired: 1 out]
                      n221 = local read "BAY 5"() -> ()  [unwired: 1 out]
                    }
                    frame Enabled {
                    }
                  }
                }
                frame #1 {
                  n222 = while {
                    tunnel: w397 -> [w400]
                    tunnel: [w399] -> w396
                    stop <- w403 stop-if-true
                    n223 = flat-sequence {
                      tunnel: [w417] -> w399
                      tunnel: w400 -> [w498]
                      tunnel: [w416] -> w398
                      frame #0 {
                        n224 = while {
                          stop <- w407 stop-if-true
                          n225 = event shown="[1] \"System Parameters Confirm Button\": Value Change" {
                            selector: _ -> [_ _]
                            dyn-events: _ -> [_ _]
                            timeout: u32 200 ("milliseconds to wait") -> [_ _]
                            tunnel: [FALSE TRUE] -> w405
                            event Timeout {
                              n226 = event-data() -> ()  [unwired: 1 in, 3 out]
                            }
                            event "System Parameters Confirm Button": Value Change {
                              n227 = event-data() -> ()  [unwired: 1 in, 5 out]
                              n228 = local write "System Parameters Confirm Button"(FALSE) -> ()
                            }
                          }
                          n229 = Wait (ms)(milliseconds to wait=u32 500) -> ()  [unwired: 1 out]
                          n230 = local read "Stop"() -> (w408:bool)
                          n231 = Or(x=w408, y=w405) -> (x .or. y?=w407:bool)
                        }
                      }
                      frame #1 {
                        w437 = 0 ("disabled index (col)")
                        w449 = 1 ("disabled index (col)")
                        # "Do while parameters have not been correctly entered"
                        n232 = local read "Bay Parameters"() -> (w436:T2)
                        n233 = local read "Synthesis Route Array"() -> (w450:string[][])
                        n234 = local read "Total Number of Experiments"() -> (w469:dbl)
                        n235 = Unbundle By Name(w436) -> ("Continue from previous optimization?"=w497:bool)
                        n236 = Unbundle By Name(w436) -> ("Excel File Name"=w499:string)
                        n237 = Unbundle By Name(w436) -> ("Matlab File"=w495:string)
                        n238 = Unbundle By Name(w436) -> ("Bay 1.Run at set flowrate"=w541:bool)
                        n239 = Unbundle By Name(w436) -> ("Bay 1.Pump 1 Flowrate"=w547:dbl)
                        n240 = Unbundle By Name(w436) -> ("Bay 1.Pump 2 Flowrate"=w546:dbl)
                        n241 = Unbundle By Name(w436) -> ("Bay 2.Run at set flowrate"=w539:bool)
                        n242 = Unbundle By Name(w436) -> ("Bay 2.Pump 3 Flowrate"=w545:dbl)
                        n243 = Unbundle By Name(w436) -> ("Bay 3.Pump 4 Flowrate"=w544:dbl)
                        n244 = Unbundle By Name(w436) -> ("Bay 3.Run at set flowrate"=w538:bool)
                        n245 = Unbundle By Name(w436) -> ("Bay 4.Run at set flowrate"=w535:bool)
                        n246 = Unbundle By Name(w436) -> ("Bay 4.Pump 5 Flowrate"=w543:dbl)
                        n247 = Unbundle By Name(w436) -> ("Bay 5.Pump 6 Flowrate"=w542:dbl)
                        n248 = Unbundle By Name(w436) -> ("Bay 5.Run at set flowrate"=w534:bool)
                        n249 = Index Array(array=w450, index (row)=3, index (col)=w449) -> (element=w443:string)
                        n250 = Index Array(array=w450, index (row)=2, index (col)=w449) -> (element=w441:string)
                        n251 = Index Array(array=w450, index (row)=1, index (col)=w449) -> (element=w439:string)
                        n252 = Index Array(array=w450, index (row)=0, index (col)=w449) -> (element=w452:string)
                        n253 = Index Array(array=w450, index (row)=4, index (col)=w449) -> (element=w445:string)
                        n254 = Index Array(array=w450, index (row)=5, index (col)=w449) -> (element=w447:string)
                        n255 = Build Array(w452, w439, w441, w443, w445, w447) -> (w453:string[])
                        n256 = Index Array(array=w450, index (row)=0 ("index"), index (col)=w437) -> (element=w475:string)
                        n257 = for {
                          tunnel: w453 -> [w549] mode=indexing
                          tunnel: [w548] -> w438 mode=indexing
                          n258 = script code="ctemp1 = str2num(c_temp);"("c_temp"=w549) -> ("ctemp1"=w548:dbl)  [unwired: 1 in, 1 out]
                        }
                        n259 = Boolean To (0,1)(Boolean=w539) -> (0, 1=w494:i16)
                        n260 = Boolean To (0,1)(Boolean=w535) -> (0, 1=w536:i16)
                        n261 = Boolean To (0,1)(Boolean=w538) -> (0, 1=w537:i16)
                        n262 = Boolean To (0,1)(Boolean=w497) -> (0, 1=w496:i16)
                        n263 = Boolean To (0,1)(Boolean=w541) -> (0, 1=w540:i16)
                        n264 = Boolean To (0,1)(Boolean=w534) -> (0, 1=w533:i16)
                        n265 = Index Array(array=w450, index (row)=1 ("index"), index (col)=w437) -> (element=w470:string)
                        n266 = Index Array(array=w450, index (row)=2 ("index"), index (col)=w437) -> (element=w471:string)
                        n267 = Unbundle By Name(w436) -> ("Bay 1.optimize_temp"=w532:bool)
                        n268 = Unbundle By Name(w436) -> ("Bay 1.optimize_tau"=w530:bool)
                        n269 = Unbundle By Name(w436) -> ("Bay 2.optimize_temp"=w528:bool)
                        n270 = Unbundle By Name(w436) -> ("Bay 2.optimize_tau"=w526:bool)
                        n271 = Unbundle By Name(w436) -> ("Bay 3.optimize_temp"=w524:bool)
                        n272 = Unbundle By Name(w436) -> ("Bay 3.optimize_tau"=w522:bool)
                        n273 = Unbundle By Name(w436) -> ("Bay 4.optimize_temp"=w520:bool)
                        n274 = Unbundle By Name(w436) -> ("Bay 4.optimize_tau"=w518:bool)
                        n275 = Index Array(array=w450, index (row)=3 ("index"), index (col)=w437) -> (element=w472:string)
                        n276 = Boolean To (0,1)(Boolean=w520) -> (0, 1=w519:i16)
                        n277 = Boolean To (0,1)(Boolean=w518) -> (0, 1=w517:i16)
                        n278 = Index Array(array=w450, index (row)=4 ("index"), index (col)=w437) -> (element=w473:string)
                        n279 = Boolean To (0,1)(Boolean=w522) -> (0, 1=w521:i16)
                        n280 = Boolean To (0,1)(Boolean=w528) -> (0, 1=w527:i16)
                        n281 = Boolean To (0,1)(Boolean=w532) -> (0, 1=w531:i16)
                        n282 = Boolean To (0,1)(Boolean=w526) -> (0, 1=w525:i16)
                        n283 = Boolean To (0,1)(Boolean=w530) -> (0, 1=w529:i16)
                        n284 = Boolean To (0,1)(Boolean=w524) -> (0, 1=w523:i16)
                        n285 = Unbundle By Name(w436) -> ("Bay 5.optimize_temp"=w516:bool)
                        n286 = Unbundle By Name(w436) -> ("Bay 5.optimize_tau"=w514:bool)
                        n287 = Index Array(array=w450, index (row)=5 ("index"), index (col)=w437) -> (element=w474:string)
                        n288 = Boolean To (0,1)(Boolean=w516) -> (0, 1=w515:i16)
                        n289 = Boolean To (0,1)(Boolean=w514) -> (0, 1=w513:i16)
                        n290 = Build Array(w531, w529, w527, w525, w523, w521, w519, w517, w515, w513) -> (w512:i16[])
                        n291 = Unbundle By Name(w436) -> ("Bay 1.Temperature Params"=w509:dbl[])
                        n292 = Unbundle By Name(w436) -> ("Bay 2.Temperature Params"=w508:dbl[])
                        n293 = Unbundle By Name(w436) -> ("Bay 2.Resisdence time params"=w503:dbl[])
                        n294 = Unbundle By Name(w436) -> ("Bay 3.Temperature Params"=w507:dbl[])
                        n295 = Unbundle By Name(w436) -> ("Bay 3.Resisdence time params"=w502:dbl[])
                        n296 = Unbundle By Name(w436) -> ("Bay 4.Temperature Params"=w506:dbl[])
                        n297 = Unbundle By Name(w436) -> ("Bay 4.Resisdence time params"=w501:dbl[])
                        n298 = Unbundle By Name(w436) -> ("Bay 5.Temperature Params"=w505:dbl[])
                        n299 = Unbundle By Name(w436) -> ("Bay 5.Resisdence time params"=w500:dbl[])
                        n300 = Unbundle By Name(w436) -> ("Bay 1.pump params 2"=w468:dbl[])
                        n301 = Unbundle By Name(w436) -> ("Bay 1.pump params 1"=w504:dbl[])
                        n302 = Unbundle By Name(w436) -> ("Bay 1.Run at set temperature"=w459:bool)
                        n303 = Unbundle By Name(w436) -> ("Bay 2.Run at set temperature"=w457:bool)
                        n304 = Unbundle By Name(w436) -> ("Bay 3.Run at set temperature"=w456:bool)
                        n305 = Unbundle By Name(w436) -> ("Bay 4.Run at set temperature"=w455:bool)
                        n306 = Unbundle By Name(w436) -> ("Bay 5.Run at set temperature"=w454:bool)
                        n307 = Unbundle By Name(w436) -> ("Bay 3.Temperature"=w465:dbl)
                        n308 = Unbundle By Name(w436) -> ("Bay 1.Temperature"=w467:dbl)
                        n309 = Unbundle By Name(w436) -> ("Bay 2.Temperature"=w466:dbl)
                        n310 = Unbundle By Name(w436) -> ("Bay 4.Temperature"=w464:dbl)
                        n311 = Unbundle By Name(w436) -> ("Bay 5.Temperature"=w463:dbl)
                        n312 = Unbundle By Name(w436) -> ("Bay 3.pump_num_ratio"=w488:dbl)
                        n313 = Unbundle By Name(w436) -> ("Bay 4.pump_num_ratio"=w485:dbl)
                        n314 = Unbundle By Name(w436) -> ("Bay 5.pump_num_ratio"=w482:dbl)
                        n315 = Unbundle By Name(w436) -> ("Bay 2.pump_num_ratio"=w491:dbl)
                        n316 = Unbundle By Name(w436) -> ("Bay 4.pump_at_ratio"=w487:bool)
                        n317 = Boolean To (0,1)(Boolean=w487) -> (0, 1=w486:i16)
                        n318 = Unbundle By Name(w436) -> ("Bay 3.pump_at_ratio"=w490:bool)
                        n319 = Boolean To (0,1)(Boolean=w490) -> (0, 1=w489:i16)
                        n320 = Unbundle By Name(w436) -> ("Bay 5.pump_at_ratio"=w484:bool)
                        n321 = Boolean To (0,1)(Boolean=w484) -> (0, 1=w483:i16)
                        n322 = Unbundle By Name(w436) -> ("Bay 2.pump_at_ratio"=w493:bool)
                        n323 = Boolean To (0,1)(Boolean=w493) -> (0, 1=w492:i16)
                        n324 = Build Array(w467, w466, w465, w464, w463) -> (w462:dbl[])
                        n325 = Build Array(w459, w457, w456, w455, w454) -> (w458:bool[])
                        n326 = local read "Syringe_pump?"() -> (w415:bool)
                        n327 = for {
                          N: 5 -> [_]
                          tunnel: w458 -> [w553] mode=indexing
                          tunnel: [w552] -> w460 mode=indexing
                          n328 = Select(t=1.0, s=w553, f=0.0) -> (s? t:f=w552:dbl)
                        }
                        n329 = Unbundle By Name(w436) -> ("Internal Standard?"=w427:bool)
                        n330 = Unbundle By Name(w436) -> ("increas_decrease_hplc_peak"=w428:bool)
                        n331 = Unbundle By Name(w436) -> ("Hplc Wait time(min)"=w420:dbl)
                        n332 = Unbundle By Name(w436) -> ("Total Number of Experiments 2"=w419:dbl)
                        n333 = Unbundle By Name(w436) -> ("hplc_start"=w424:dbl)
                        n334 = Unbundle By Name(w436) -> ("ISTD start"=w422:dbl)
                        n335 = Unbundle By Name(w436) -> ("hplc_end"=w423:dbl)
                        n336 = Unbundle By Name(w436) -> ("throughput_yield"=w429:bool)
                        n337 = Unbundle By Name(w436) -> ("ISTD end"=w421:dbl)
                        n338 = Select(t=1.0, s=w415, f=0.0) -> (s? t:f=w414:dbl)
                        n339 = Select(t=1.0, s=w428, f=0.0) -> (s? t:f=w426:dbl)
                        n340 = Select(t=1.0, s=w427, f=0.0) -> (s? t:f=w425:dbl)
                        n341 = Select(t=0.0, s=w429, f=1.0) -> (s? t:f=w418:dbl)
                        n342 = script code="system_error = 0;\nnumPeaks = 1;\nstart_phase_time = 1;\nis_redo_exp = 0;\nfbest_prev = 0;\nxbest_prev = [];\nFvalues = [];\nHPLC_Area = [];\n\nT1_span = [1 1]; T2_span = [1 1]; T3_span = [1 1]; T4_span = [1 1]; T5_span = [1 1];\nT_span = [T1_span;T2_span;T3_span;T4_span;T5_span];\n p1_span =  [1 1]; p2_span =  [1 1]; p3_span =  [1 1]; p4_span =  [1 1]; p5_span =  [1 1];  p6_span =  [1 1];\nOpt_params = [0 0 0 0 0 0 0 0 0 0 0];\nT_params = [T1_params;T2_params;T3_params;T4_params;T5_params];\npump_params = [pump1_params;pump2_params;pump3_params;pump4_params;pump5_params;pump6_params];\nopt_ctr = 0;ncall = 100;record_data = true;\nT1_SP = 23; T2_SP = 23; T3_SP = 23; T4_SP = 23; T5_SP = 23;\nT_span = [T1_span;T2_span;T3_span;T4_span;T5_span];\np_span = [p1_span;p2_span;p3_span;p4_span;p5_span;p6_span];\nno_errors = 1;\nP1 = 0; P2 =0; P3 = 0; P4 = 0; P5 = 0; P6 = 0;\nP = [P1, P2, P3,P4, P5, P6];\nis_first_set_of_exp = true;\nerror_message = 'System has no errors to report';\naddpath(genpath('C:\\Users\\HPLC\\Dropbox (MIT)\\MoD Files\\MATLAB'))\n%addpath(genpath('C:\\Users\\Admin\\Dropbox (MIT)\\MoD Files\\MATLAB'))\nallMSData = [];allHPLCData = [];allHPLCFile = [];\nBay_ratio = [0,Bay2_ratio,Bay3_ratio,Bay4_ratio,Bay5_ratio];\nBay_pump_ratio = [1, Bay2_pump_ratio, Bay3_pump_ratio, Bay4_pump_ratio, Bay5_pump_ratio];\nP_setrate = [P1_setrate, P2_setrate, P3_setrate, P4_setrate, P5_setrate, P6_setrate];\nuse_flowrate = [use_flowrate1, use_flowrate2,use_flowrate3, use_flowrate4, use_flowrate5];\npump_chem_name= []\nCurrExp = 1;\n% ****************************************************************************************************\n%Setup optimization\n   setup_optimization_params;\n   initialize_opt = 0;\n   nstop0 = 0;\n%*****************************************************************************************************\n% Setup excel and xml file writing\npath(path, pa);\nnumMSSig = 1;\nsetup_excel_output;\n%***************************************************************************************************\nredo = false;\nncall = ncall_in;"("use_flowrate1"=w540, "P1_setrate"=w547, "P2_setrate"=w546, "P3_setrate"=w545, "P4_setrate"=w544, "P5_setrate"=w543, "P6_setrate"=w542, "use_flowrate2"=w494, "use_flowrate3"=w537, "use_flowrate4"=w536, "use_flowrate5"=w533, "Optimize_params"=w512, "T1_params"=w509, "T2_params"=w508, "T3_params"=w507, "T4_params"=w506, "T5_params"=w505, "pump1_params"=w504, "pump3_params"=w503, "pump4_params"=w502, "pump5_params"=w501, "pump6_params"=w500, "xl_file"=w499, "pa"=w498, "Continue"=w496, "matlabsavefile"=w495, "Bay2_ratio"=w492, "Bay2_pump_ratio"=w491, "Bay3_ratio"=w489, "Bay3_pump_ratio"=w488, "Bay4_ratio"=w486, "Bay4_pump_ratio"=w485, "Bay5_ratio"=w483, "Bay5_pump_ratio"=w482, "pump1_chem"=w475, "pump6_chem"=w474, "pump5_chem"=w473, "pump4_chem"=w472, "pump3_chem"=w471, "pump2_chem"=w470, "Pump_concen"=w438, "ncall_in"=w469, "pump2_params"=w468, "T_SP"=w462, "Run_at_T_SP"=w460, "dcr_hplc_peak"=w426, "use_internal_std"=w425, "hplc_peak_start"=w424, "hplc_peak_end"=w423, "ISTD_start"=w422, "ISTD_end"=w421, "hplc_wait_time"=w420, "tot_num_exp"=w419, "throughput_yield"=w418, "syringe_pump"=w414) -> ("no_errors"=w511:dbl, "error_message"=w510:string)  [unwired: 1 in, 1 out]
                        n343 = Not Equal To 0?(x=w511) -> (x != 0?=w416:bool)
                        n344 = Not(x=w416) -> (.not. x?=w417:bool)
                        n345 = case shown="False" w417 {
                          tunnel: w510 -> [_ w555]
                          frame False {
                            n346 = local write "Setup Confirm 2"(TRUE ("Setup Confirm 2")) -> ()
                          }
                          frame True {
                            n347 = One Button Dialog(message=w555) -> ()  [unwired: 1 in, 1 out]
                          }
                        }
                      }
                    }
                    n348 = local read "Stop"() -> (w402:bool)
                    n349 = Or(x=w398, y=w402) -> (x .or. y?=w403:bool)
                    n350 = Wait (ms)(milliseconds to wait=u32 500) -> ()  [unwired: 1 out]
                  }
                }
                frame #2 {
                  n351 = local write "System Error"(w556) -> ()
                }
              }
            }
          }
        }
        frame #2 {
          # "Run Initial diagnostics"
        }
        frame #3 {
          # "Run System"
          n352 = while {
            stop <- w1167 stop-if-true
            n353 = local read "running?"() -> (w1164:bool)
            n354 = local read "Temperature Control 1"() -> (w1165:bool)
            n355 = And(x=w1164, y=w1165) -> (x .and. y?=w1161:bool)
            n356 = And(x=w1161, y=FALSE) -> (x .and. y?=w1162:bool)
            n357 = case shown="True" w1162 {
              frame False {
                n358 = local write "Temp SS? 1"(TRUE ("Temp SS? 1")) -> ()
              }
              frame True {
                # "Bay 1 Temperature Controller"
                n359 = local read "Temperature SP 1"() -> (w1169:dbl)
                n360 = local read "Temperature 1"() -> (w1173:dbl)
                n361 = local read "SSR Duration 1"() -> (w1188:dbl)
                n362 = call-poly <vilib>:"PID Online Autotuning.vi"("setpoint"=w1169, "manipulated variable"=w1188, "autotuning parameters"=T9 {"type of controller"=enum."PID", "relay cycles"=3, "relay amplitude"=1.0, "control specifications"=enum."Normal", "PV noise level"=0.1} ("Autotuning Parameters R1"), "process variable"=w1173, "PID gains in"=T8 {"Proportional gain Kc"=0.38538, "Integral time Ti (sec)"=0.524375, "Derivative time Ti (sec)"=0.12585} ("PID gains 2")) -> ("setpoint out"=w1194:dbl, "process variable out"=w1193:dbl, "PID gains out"=w1190:T11)  [unwired: 6 in, 2 out]
                n363 = call <vilib>:"PID Autotuning (Temperature).vi"("desired temperature"=w1194, "measured temperature"=w1193, "plant parameters in"=w1190, "output range"=cluster{"output high":dbl, "output low":dbl} {"output high"=3.0, "output low"=-1.0} ("Output range")) -> ("output"=w1186:dbl)  [unwired: 12 in, 3 out]
                n364 = local write "SSR Duration 1"(w1186) -> ()
                n365 = Subtract(x=w1169, y=w1173) -> (x-y=w1180:dbl)
                n366 = Absolute Value(x=w1180) -> (abs(x)=w1183:dbl)
                n367 = Multiply(x=1000.0, y=w1186) -> (x*y=w1184:dbl)
                n368 = Greater Than 0?(x=w1184) -> (x > 0?=w1178:bool)
                n369 = Less Or Equal?(x=w1183, y=1.2) -> (x <= y?=w1181:bool)
                n370 = Greater?(x=w1169, y=w1173) -> (0:w1179:bool)
                n371 = And(x=w1178, y=w1179) -> (x .and. y?=w1176:bool)
                n372 = local write "Temp SS? 1"(w1181) -> ()
                n373 = Subtract(x=w1173, y=10.0) -> (x-y=w1174:dbl)
                n374 = Less?(x=w1174, y=w1169) -> (x < y?=w1177:bool)
                n375 = And(x=w1177, y=w1176) -> (x .and. y?=w1175:bool)
                n376 = case shown="True" w1175 {
                  tunnel: [errorcluster {"status"=FALSE, "code"=0, "source"=""} ("error out") w1203] -> _
                  tunnel: 2 -> [_ w1201]
                  tunnel: w1184 -> [w1198 w1202]
                  tunnel: [0.0 w1205] -> w1171
                  tunnel: w1169 -> [_ w1204]
                  frame False {
                    n377 = Absolute Value(x=w1198) -> (abs(x)=w1199:dbl)
                    n378 = Wait (ms)(milliseconds to wait=w1199) -> ()  [unwired: 1 out]
                  }
                  frame True {
                    n379 = call "TurnOnRelayArduino.vi"("channel"=w1201, "duration"=w1202) -> ("error out"=w1203:errorcluster)  [unwired: 8 in, 1 out]
                    n380 = script code="tempdiff1= SP1 - T1;\nif tempdiff1 > 10\n  if slope1 < .01\n     temp_check1 = temp_check1 + 1;\n  else\n      temp_check1 =0;\n  end\nend\n\nif temp_check1 > 9\n  temp_error1 = 1\nend"("SP1"=w1204) -> ("temp_error1"=w1205:dbl)  [unwired: 1 in, 1 out]
                  }
                }
                n381 = Not Equal To 0?(x=w1171) -> (x != 0?=w1170:bool)
                n382 = case shown="True" w1170 {
                  frame False {
                  }
                  frame True {
                    n383 = local write "Error Message"("Bay 1 Temperature Heating Error") -> ()
                  }
                }
                n384 = case shown="True" w1170 {
                  tunnel: w1170 -> [_ w1196]
                  frame False {
                  }
                  frame True {
                    n385 = local write "System Error"(w1196) -> ()
                    n386 = local write "Stop"(w1196) -> ()
                  }
                }
              }
            }
            n387 = Wait (ms)(milliseconds to wait=u32 400) -> ()  [unwired: 1 out]
            n388 = local read "Stop"() -> (w1167:bool)
          }
          n389 = local read "Bay Parameters"() -> (w559:T2)
          n390 = while {
            stop <- w1122 stop-if-true
            n391 = local read "running?"() -> (w1119:bool)
            n392 = local read "Temperature Control 2"() -> (w1120:bool)
            n393 = And(x=w1119, y=w1120) -> (x .and. y?=w1116:bool)
            n394 = local read "Stop"() -> (w1122:bool)
            n395 = Wait (ms)(milliseconds to wait=u32 400) -> ()  [unwired: 1 out]
            n396 = And(x=w1116, y=FALSE) -> (x .and. y?=w1118:bool)
            n397 = case shown="True" w1118 {
              frame False {
                n398 = local write "Temp SS? 2"(TRUE ("Temp SS? 2")) -> ()
              }
              frame True {
                # "Bay 2 Temperature Controller"
                n399 = local read "Temperature SP 2"() -> (w1125:dbl)
                n400 = local read "Temperature 2"() -> (w1128:dbl)
                n401 = local read "SSR Duration 2"() -> (w1146:dbl)
                n402 = call-poly <vilib>:"PID Online Autotuning.vi"("setpoint"=w1125, "manipulated variable"=w1146, "autotuning parameters"=T9 {"type of controller"=enum."PID", "relay cycles"=3, "relay amplitude"=1.0, "control specifications"=enum."Normal", "PV noise level"=0.1} ("Autotuning Parameters R1"), "process variable"=w1128, "PID gains in"=T8 {"Proportional gain Kc"=0.38538, "Integral time Ti (sec)"=0.524375, "Derivative time Ti (sec)"=0.12585} ("PID gains 2")) -> ("setpoint out"=w1144:dbl, "process variable out"=w1143:dbl, "PID gains out"=w1149:T11)  [unwired: 6 in, 2 out]
                n403 = call <vilib>:"PID Autotuning (Temperature).vi"("desired temperature"=w1144, "measured temperature"=w1143, "plant parameters in"=w1149, "output range"=cluster{"output high":dbl, "output low":dbl} {"output high"=3.0, "output low"=-1.0} ("Output range")) -> ("output"=w1139:dbl)  [unwired: 12 in, 3 out]
                n404 = local write "SSR Duration 2"(w1139) -> ()
                n405 = Greater?(x=w1125, y=w1128) -> (0:w1134:bool)
                n406 = Multiply(x=1000.0, y=w1139) -> (x*y=w1141:dbl)
                n407 = Greater Than 0?(x=w1141) -> (x > 0?=w1133:bool)
                n408 = And(x=w1133, y=w1134) -> (x .and. y?=w1131:bool)
                n409 = Subtract(x=w1125, y=w1128) -> (x-y=w1136:dbl)
                n410 = Absolute Value(x=w1136) -> (abs(x)=w1138:dbl)
                n411 = Subtract(x=w1128, y=10.0) -> (x-y=w1130:dbl)
                n412 = Less Or Equal?(x=w1138, y=1.2) -> (x <= y?=w1135:bool)
                n413 = local write "Temp SS? 2"(w1135) -> ()
                n414 = Less?(x=w1130, y=w1125) -> (x < y?=w1132:bool)
                n415 = And(x=w1132, y=w1131) -> (x .and. y?=w1127:bool)
                n416 = case shown="True" w1127 {
                  tunnel: [errorcluster {"status"=FALSE, "code"=0, "source"=""} ("error out") w1158] -> _
                  tunnel: 3 -> [_ w1156]
                  tunnel: w1141 -> [w1153 w1157]
                  tunnel: [0.0 w1160] -> w1126
                  tunnel: w1125 -> [_ w1159]
                  frame False {
                    n417 = Absolute Value(x=w1153) -> (abs(x)=w1154:dbl)
                    n418 = Wait (ms)(milliseconds to wait=w1154) -> ()  [unwired: 1 out]
                  }
                  frame True {
                    n419 = call "TurnOnRelayArduino.vi"("channel"=w1156, "duration"=w1157) -> ("error out"=w1158:errorcluster)  [unwired: 8 in, 1 out]
                    n420 = script code="tempdiff2= SP2 - T2;\nif tempdiff2 > 10\n  if slope2 < .01\n     temp_check2 = temp_check2 + 1;\n  else\n      temp_check2 =0;\n  end\nend\n\nif temp_check2 > 9\n  temp_error2 = 1\nend"("SP2"=w1159) -> ("temp_error2"=w1160:dbl)  [unwired: 1 in, 1 out]
                  }
                }
                n421 = Not Equal To 0?(x=w1126) -> (x != 0?=w1124:bool)
                n422 = case shown="True" w1124 {
                  frame False {
                  }
                  frame True {
                    n423 = local write "Error Message"("Bay 2 Temperature Heating Error") -> ()
                  }
                }
                n424 = case shown="True" w1124 {
                  tunnel: w1124 -> [_ w1151]
                  frame False {
                  }
                  frame True {
                    n425 = local write "Stop"(w1151) -> ()
                    n426 = local write "System Error"(w1151) -> ()
                  }
                }
              }
            }
          }
          n427 = local read "Stop"() -> (w557:bool)
          n428 = Not(x=w557) -> (.not. x?=w558:bool)
          n429 = case shown="True" w558 {
            tunnel: w559 -> [_ w562]
            frame False {
            }
            frame True {
              n430 = while {
                tunnel: w562 -> [w574]
                i -> [w573]
                stop <- w567 stop-if-true
                n431 = local read "running?"() -> (w563:bool)
                n432 = Wait (ms)(milliseconds to wait=u32 1000) -> ()  [unwired: 1 out]
                n433 = Increment(x=w573) -> (x+1=w564:i32)
                n434 = case shown="True" w563 {
                  tunnel: w573 -> [w579 _]
                  tunnel: w574 -> [_ _]
                  tunnel: [w581 w582] -> w565
                  tunnel: [0.0 w583] -> w569
                  frame False {
                    # "STANDBY MODE"
                    n435 = Add(x=w579, y=2.0) -> (x+y=w581:dbl)
                  }
                  frame True {
                    n436 = flat-sequence {
                      tunnel: [w593] -> w583
                      tunnel: [200.0] -> w582
                      frame #0 {
                        n437 = local write "stop_xl_write"(FALSE ("stop_xl_write")) -> ()
                      }
                      frame #1 {
                        # "Increase flowrate of dilution stream"
                        # "Wait mixed stream reaches SL"
                        # "SNOBFIT"
                        # "Optimize"
                        # "Run Experimental Conditions"
                        # "Optimize/Synthesize"
                        n438 = local read "Syringe_pump?"() -> (w586:bool)
                        n439 = local read "Stop"() -> (w589:bool)
                        n440 = Not(x=w589) -> (.not. x?=w588:bool)
                        n441 = case shown="True" w588 {
                          tunnel: [1.0 w615] -> w596
                          tunnel: [w603 w614] -> w591
                          tunnel: [0.0 w613] -> w590
                          tunnel: [w603 w612] -> w587
                          tunnel: w586 -> [_ w609]
                          frame False {
                            w603 = dbl[] []
                          }
                          frame True {
                            n442 = Select(t=1.0, s=w609, f=0.0) -> (s? t:f=w608:dbl)
                            n443 = script code="optimization_main_loop_epox_additives"("syringe_pump"=w608) -> ("Conditions_Array"=w614:dbl[], "opt_ctr"=w615:dbl, "P_tot"=w613:dbl, "tau_array"=w612:dbl[], "experiment_history"=w610:dbl[][])  [unwired: 1 in, 1 out]
                            n444 = call-poly <vilib>:"Array To Matrix.vi"("Real 2D Array"=w610) -> ("Real Matrix"=w611:T12)
                            n445 = local write "experiment history"(w611) -> ()
                          }
                        }
                        "P_tot" <- w590
                        n446 = local read "COMM Port :: Milligat Pumps"() -> (w597:refnum<visa-resource-name>)
                        n447 = Equal?(x=w596, y=1.0) -> (x = y?=w594:bool)
                        n448 = flat-sequence {
                          tunnel: w591 -> [w964]
                          tunnel: w587 -> [w958]
                          frame #0 {
                            # "Start recording data"
                            n449 = Index Array(array=w964, index=5) -> (element=w976:dbl)
                            n450 = Index Array(array=w964, index=0) -> (element=w971:dbl)
                            n451 = Index Array(array=w964, index=1) -> (element=w972:dbl)
                            n452 = Index Array(array=w964, index=2) -> (element=w974:dbl)
                            n453 = Index Array(array=w964, index=3) -> (element=w973:dbl)
                            n454 = Index Array(array=w964, index=4) -> (element=w975:dbl)
                            n455 = local write "Pump setpoint(ul/min) 2"(w972) -> ()
                            n456 = local write "Pump setpoint(ul/min) 4"(w974) -> ()
                            n457 = local write "Pump setpoint(ul/min) 5"(w975) -> ()
                            n458 = local write "Pump setpoint(ul/min) 3"(w973) -> ()
                            n459 = local write "Pump setpoint(ul/min) 6"(w976) -> ()
                            n460 = local write "Pump setpoint(ul/min) 1"(w971) -> ()
                            n461 = Index Array(array=w958, index=0) -> (element=w963:dbl)
                            n462 = Index Array(array=w958, index=4) -> (element=w962:dbl)
                            n463 = Index Array(array=w958, index=3) -> (element=w961:dbl)
                            n464 = Index Array(array=w958, index=2) -> (element=w960:dbl)
                            n465 = Index Array(array=w958, index=1) -> (element=w959:dbl)
                            n466 = local write "tau 2"(w959) -> ()
                            n467 = local write "tau 3"(w960) -> ()
                            n468 = local write "tau 4"(w961) -> ()
                            n469 = local write "tau 5"(w962) -> ()
                            n470 = local write "tau 1"(w963) -> ()
                          }
                        }
                        n471 = flat-sequence {
                          tunnel: w597 -> [w619]
                          tunnel: w591 -> [w618]
                          tunnel: w594 -> [w617]
                          tunnel: [w617] -> w602
                          tunnel: w602 -> [w764]
                          tunnel: [w764] -> w601
                          tunnel: w601 -> [w784]
                          tunnel: [w782] -> w585
                          tunnel: w591 -> [w807]
                          tunnel: w585 -> [w806]
                          tunnel: [w897] -> w600
                          tunnel: w600 -> [w910]
                          tunnel: [w910] -> w599
                          tunnel: w599 -> [w918]
                          tunnel: [w918] -> w598
                          tunnel: [w952] -> w593
                          tunnel: w598 -> [w952]
                          frame #0 {
                            # "Setup pump flowrates and temperature setpoints"
                            n472 = local read "Pump Addresses"() -> (w616:string[])
                            n473 = stacked-sequence {
                              tunnel: w619 -> [w642 _ _ _ _]
                              tunnel: w619 -> [_ w679 _ _ _]
                              tunnel: w619 -> [_ _ w707 _ _]
                              tunnel: w619 -> [_ _ _ w732 _]
                              tunnel: w619 -> [_ _ _ _ w757]
                              tunnel: w618 -> [w639 w677 w705 w730 w754]
                              tunnel: w617 -> [w629 w670 w700 w723 w748]
                              tunnel: w616 -> [w620 w662 w687 w715 w740]
                              frame #0 {
                                # "Bay 1"
                                n474 = local read "Syringe_pump?"() -> (w628:bool)
                                n475 = Index Array(array=w639, index=0) -> (element=w637:dbl)
                                n476 = local read "BAY 1"() -> (w623:u16)
                                n477 = Index Array(array=w639, index=1) -> (element=w636:dbl)
                                n478 = Index Array(array=w639, index=6) -> (element=w635:dbl)
                                n479 = script code="MATLAB script"("T1_SP"=w635) -> ()  [unwired: 1 in, 1 out]
                                n480 = Less Or Equal?(x=w623, y=u16 4) -> (x <= y?=w625:bool)
                                n481 = Greater Or Equal?(x=w623, y=u16 1) -> (x >= y?=w626:bool)
                                n482 = And(x=w626, y=w625) -> (x .and. y?=w627:bool)
                                n483 = Greater Than 0?(x=w637) -> (x > 0?=w634:bool)
                                n484 = And(x=w634, y=w629) -> (x .and. y?=w633:bool)
                                n485 = Greater Than 0?(x=w636) -> (x > 0?=w632:bool)
                                n486 = Wait (ms)(milliseconds to wait=u32 300) -> ()  [unwired: 1 out]
                                n487 = And(x=w632, y=w629) -> (x .and. y?=w631:bool)
                                n488 = And(x=w627, y=w629) -> (x .and. y?=w630:bool)
                                n489 = case shown="False" w628 {
                                tunnel: w642 -> [w646 _]
                                tunnel: w636 -> [w645 w653]
                                tunnel: w631 -> [w644 w654]
                                tunnel: w620 -> [w643 _]
                                frame False {
                                n490 = case shown="True" w644 {
                                tunnel: w646 -> [w649 _]
                                tunnel: w645 -> [_ _]
                                tunnel: w643 -> [w648 w652]
                                frame False {
                                n491 = Index Array(array=w648, index=1) -> (element=w650:string)
                                n492 = call "PumpStop.vi"("Pump Address"=w650, "Pump COMM Port"=w649) -> ()  [unwired: 9 in, 1 out]
                                }
                                frame True {
                                n493 = Index Array(array=w652, index=1) -> ()  [unwired: 1 out]
                                }
                                }
                                }
                                frame True {
                                n494 = case shown="True" w654 {
                                tunnel: w653 -> [_ _]
                                frame False {
                                }
                                frame True {
                                }
                                }
                                }
                                }
                                n495 = case shown="False" w633 {
                                tunnel: w642 -> [_ _]
                                tunnel: w637 -> [_ _]
                                tunnel: w620 -> [w659 w661]
                                frame False {
                                n496 = Index Array(array=w659, index=0) -> ()  [unwired: 1 out]
                                }
                                frame True {
                                n497 = Index Array(array=w661, index=0) -> ()  [unwired: 1 out]
                                }
                                }
                                n498 = case shown="True" w630 {
                                tunnel: w635 -> [_ w657]
                                frame False {
                                n499 = local write "Temperature Control 1"(FALSE) -> ()
                                }
                                frame True {
                                n500 = local write "Temperature SP 1"(w657) -> ()
                                n501 = local write "Temperature Control 1"(TRUE ("Temperature Control 1")) -> ()
                                }
                                }
                              }
                              frame #1 {
                                # "Bay 2"
                                n502 = local read "BAY 2"() -> (w666:u16)
                                n503 = Index Array(array=w677, index=2) -> (element=w674:dbl)
                                n504 = Index Array(array=w677, index=7) -> (element=w675:dbl)
                                n505 = script code="MATLAB script"("T2_SP"=w675) -> ()  [unwired: 1 in, 1 out]
                                n506 = Greater Than 0?(x=w674) -> (x > 0?=w672:bool)
                                n507 = And(x=w672, y=w670) -> (x .and. y?=w671:bool)
                                n508 = Greater Or Equal?(x=w666, y=u16 1) -> (x >= y?=w664:bool)
                                n509 = Less Or Equal?(x=w666, y=u16 4) -> (x <= y?=w669:bool)
                                n510 = And(x=w664, y=w669) -> (x .and. y?=w668:bool)
                                n511 = And(x=w668, y=w670) -> (x .and. y?=w673:bool)
                                n512 = case shown="True" w673 {
                                tunnel: w675 -> [_ w685]
                                frame False {
                                n513 = local write "Temperature Control 2"(FALSE) -> ()
                                }
                                frame True {
                                n514 = local write "Temperature Control 2"(TRUE ("Temperature Control 2")) -> ()
                                n515 = local write "Temperature SP 2"(w685) -> ()
                                }
                                }
                                n516 = case shown="False" w671 {
                                tunnel: w674 -> [_ _]
                                tunnel: w679 -> [_ _]
                                tunnel: w662 -> [w680 w682]
                                frame False {
                                n517 = Index Array(array=w680, index=2) -> ()  [unwired: 1 out]
                                }
                                frame True {
                                n518 = Index Array(array=w682, index=2) -> ()  [unwired: 1 out]
                                }
                                }
                                n519 = Wait (ms)(milliseconds to wait=u32 300) -> ()  [unwired: 1 out]
                              }
                              frame #2 {
                                # "Bay 3"
                                n520 = local read "BAY 3"() -> (w695:u16)
                                n521 = Index Array(array=w705, index=3) -> (element=w703:dbl)
                                n522 = Not Equal To 0?(x=w703) -> (x != 0?=w702:bool)
                                n523 = Index Array(array=w705, index=8) -> (element=w690:dbl)
                                n524 = script code="MATLAB script"("T3_SP"=w690) -> ()  [unwired: 1 in, 1 out]
                                n525 = Less Or Equal?(x=w695, y=u16 4) -> (x <= y?=w699:bool)
                                n526 = Greater Or Equal?(x=w695, y=u16 1) -> (x >= y?=w696:bool)
                                n527 = And(x=w696, y=w699) -> (x .and. y?=w694:bool)
                                n528 = And(x=w694, y=w700) -> (x .and. y?=w692:bool)
                                n529 = And(x=w702, y=w700) -> (x .and. y?=w701:bool)
                                n530 = Not Equal?(x=w690, y=23.0) -> (x != y?=w691:bool)
                                n531 = And(x=w692, y=w691) -> (x .and. y?=w688:bool)
                                n532 = case shown="True" w701 {
                                tunnel: w703 -> [_ _]
                                tunnel: w707 -> [_ _]
                                tunnel: w687 -> [w708 w710]
                                frame False {
                                n533 = Index Array(array=w708, index=3) -> ()  [unwired: 1 out]
                                }
                                frame True {
                                n534 = Index Array(array=w710, index=3) -> ()  [unwired: 1 out]
                                }
                                }
                                n535 = case shown="True" w688 {
                                tunnel: w690 -> [_ w713]
                                frame False {
                                n536 = local write "Temperature Control 3"(FALSE) -> ()
                                }
                                frame True {
                                n537 = local write "Temperature Control 3"(TRUE ("Temperature Control 3")) -> ()
                                n538 = local write "Temperature SP 3"(w713) -> ()
                                }
                                }
                                n539 = Wait (ms)(milliseconds to wait=u32 300) -> ()  [unwired: 1 out]
                              }
                              frame #3 {
                                # "Bay 4"
                                n540 = Index Array(array=w730, index=9) -> (element=w727:dbl)
                                n541 = script code="MATLAB script"("T4_SP"=w727) -> ()  [unwired: 1 in, 1 out]
                                n542 = Index Array(array=w730, index=4) -> (element=w728:dbl)
                                n543 = Not Equal To 0?(x=w728) -> (x != 0?=w726:bool)
                                n544 = local read "BAY 4"() -> (w717:u16)
                                n545 = And(x=w726, y=w723) -> (x .and. y?=w725:bool)
                                n546 = Less Or Equal?(x=w717, y=u16 4) -> (x <= y?=w722:bool)
                                n547 = Greater Or Equal?(x=w717, y=u16 1) -> (x >= y?=w719:bool)
                                n548 = And(x=w719, y=w722) -> (x .and. y?=w718:bool)
                                n549 = And(x=w718, y=w723) -> (x .and. y?=w724:bool)
                                n550 = case shown="False" w725 {
                                tunnel: w732 -> [_ _]
                                tunnel: w728 -> [_ _]
                                tunnel: w715 -> [w733 w735]
                                frame False {
                                n551 = Index Array(array=w733, index=4) -> ()  [unwired: 1 out]
                                }
                                frame True {
                                n552 = Index Array(array=w735, index=4) -> ()  [unwired: 1 out]
                                }
                                }
                                n553 = case shown="True" w724 {
                                tunnel: w727 -> [_ w738]
                                frame False {
                                n554 = local write "Temperature Control 4"(FALSE ("Temperature Control 4")) -> ()
                                }
                                frame True {
                                n555 = local write "Temperature SP 4"(w738) -> ()
                                n556 = local write "Temperature Control 4"(TRUE ("Temperature Control 5")) -> ()
                                }
                                }
                                n557 = Wait (ms)(milliseconds to wait=u32 300) -> ()  [unwired: 1 out]
                              }
                              frame #4 {
                                # "Bay 5"
                                n558 = Index Array(array=w754, index=5) -> (element=w752:dbl)
                                n559 = Index Array(array=w754, index=4) -> (element=w753:dbl)
                                n560 = script code="MATLAB script"("T5_SP"=w753) -> ()  [unwired: 1 in, 1 out]
                                n561 = local read "BAY 5"() -> (w743:u16)
                                n562 = Not Equal To 0?(x=w752) -> (x != 0?=w750:bool)
                                n563 = And(x=w750, y=w748) -> (x .and. y?=w749:bool)
                                n564 = Less Or Equal?(x=w743, y=u16 4) -> (x <= y?=w747:bool)
                                n565 = Greater Or Equal?(x=w743, y=u16 1) -> (x >= y?=w744:bool)
                                n566 = case shown="True" w749 {
                                tunnel: w757 -> [_ _]
                                tunnel: w752 -> [_ _]
                                tunnel: w740 -> [w758 _]
                                frame False {
                                n567 = Index Array(array=w758, index=5) -> ()  [unwired: 1 out]
                                }
                                frame True {
                                (unwired) 5 ("index")
                                }
                                }
                                n568 = And(x=w744, y=w747) -> (x .and. y?=w742:bool)
                                n569 = And(x=w742, y=w748) -> (x .and. y?=w751:bool)
                                n570 = case shown="False" w751 {
                                tunnel: w753 -> [_ w761]
                                frame False {
                                n571 = local write "Temperature Control 5"(FALSE ("Temperature Control 5")) -> ()
                                }
                                frame True {
                                n572 = local write "Temperature SP 5"(w761) -> ()
                                n573 = local write "Temperature Control 5"(TRUE ("Temperature Control 5")) -> ()
                                }
                                }
                                n574 = Wait (ms)(milliseconds to wait=u32 300) -> ()  [unwired: 1 out]
                              }
                            }
                          }
                          frame #1 {
                            # "Wait till Steady State temperature readings on all bays"
                            n575 = while {
                              tunnel: w764 -> [w765]
                              stop <- w766 stop-if-true
                              n576 = flat-sequence {
                                tunnel: [w769] -> w766
                                tunnel: w765 -> [w768]
                                frame #0 {
                                n577 = Wait (ms)(milliseconds to wait=u32 1500) -> ()  [unwired: 1 out]
                                }
                                frame #1 {
                                n578 = local read "Temp SS? 2"() -> (w772:bool)
                                n579 = local read "Temp SS? 3"() -> (w773:bool)
                                n580 = local read "Temp SS? 4"() -> (w774:bool)
                                n581 = local read "Temp SS? 5"() -> (w775:bool)
                                n582 = local read "Temp SS? 1"() -> (w771:bool)
                                n583 = Not(x=w768) -> (.not. x?=w781:bool)
                                n584 = local read "Stop"() -> (w770:bool)
                                n585 = And(x=w773, y=w774) -> (x .and. y?=w777:bool)
                                n586 = And(x=w771, y=w772) -> (x .and. y?=w778:bool)
                                n587 = And(x=w778, y=w777) -> (x .and. y?=w776:bool)
                                n588 = And(x=w776, y=w775) -> (x .and. y?=w779:bool)
                                n589 = Or(x=w781, y=w779) -> (x .or. y?=w780:bool)
                                n590 = Or(x=w780, y=w770) -> (x .or. y?=w769:bool)
                                }
                              }
                            }
                            n591 = local write "Calculate condition"(TRUE ("Calculate condition")) -> ()
                          }
                          frame #2 {
                            n592 = flat-sequence {
                              tunnel: w784 -> [w786]
                              tunnel: [w786] -> w783
                              tunnel: w783 -> [w793]
                              tunnel: [w793] -> w782
                              frame #0 {
                                n593 = local write "Equlibrating Temperature"(TRUE) -> ()
                              }
                              frame #1 {
                                # "Wait 2.5 system volumes"
                                n594 = local read "Number of System Flushes per condtion"() -> (w790:dbl)
                                n595 = local read "Extra system dead volume"() -> (w791:dbl)
                                n596 = script code="start = tic;\nP_tot = P1+P2+P3+P4+P5+P6;\nif P_tot >0\n  extra_res = extr_sys_dead_vol/P_tot;\nelse\n   extra_res =0;\nend\ntotal_sys_res = tau1 + tau2 + tau3 + tau4 + tau5 + extra_res;\ntotal_wait_time = 15;"("extr_sys_dead_vol"=w791, "num_flush_per_cond"=w790) -> ("??"=w794:errorcluster, "total_wait_time"=w788:dbl, "total_sys_res"=→"Total System Resisdence Time(min)":dbl)  [unwired: 1 in]
                                n597 = Divide(x=w788, y=60.0) -> (x/y=→"total_flush_time":dbl)
                                n598 = while {
                                tunnel: w793 -> [w796]
                                tunnel: w794 -> [w799]
                                stop <- w800 stop-if-true
                                # "Check if system is flushed every 5 seconds"
                                n599 = script code="end1 = toc(start);\nflush_time = 0;\nif end1 > total_wait_time\n   flush_time = 1;\nend\ncurr_wait_time = end1 /60;"("??"=w799) -> ("flush_time"=w803:dbl, "curr_wait_time"=w798:dbl)  [unwired: 1 out]
                                "curr_wait_time" <- w798
                                n600 = Not Equal To 0?(x=w803) -> (x != 0?=w802:bool)
                                n601 = Multiply(x=60.0, y=w798) -> ()  [unwired: 1 out]
                                n602 = local read "Stop"() -> (w805:bool)
                                n603 = Or(x=w802, y=w805) -> (x .or. y?=w801:bool)
                                n604 = Not(x=w796) -> (.not. x?=w795:bool)
                                n605 = Wait (ms)(milliseconds to wait=u32 5000) -> ()  [unwired: 1 out]
                                n606 = Or(x=w801, y=w795) -> (x .or. y?=w800:bool)
                                }
                              }
                            }
                          }
                          frame #3 {
                            # "Collect HPLC Data"
                            n607 = flat-sequence {
                              tunnel: w807 -> [w812]
                              tunnel: w806 -> [w811]
                              frame #0 {
                                n608 = local read "pause for ms"() -> (w810:bool)
                                n609 = case shown="True" w810 {
                                frame False {
                                }
                                frame True {
                                }
                                }
                                n610 = local write "Flushing System"(TRUE ("Flushing System")) -> ()
                                "System Flushed?" <- TRUE ("System Flushed?")
                              }
                              frame #1 {
                                n611 = flat-sequence {
                                tunnel: w812 -> [w814]
                                tunnel: w811 -> [_]
                                frame #0 {
                                }
                                frame #1 {
                                n612 = flat-sequence {
                                tunnel: w814 -> [w815]
                                tunnel: w814 -> [_]
                                tunnel: [w866] -> w813
                                tunnel: w813 -> [_]
                                frame #0 {
                                n613 = local read "COMM Port :: Milligat Pumps"() -> (w817:refnum<visa-resource-name>)
                                n614 = stacked-sequence {
                                tunnel: w817 -> [w820 w829 w838 w840 w846 w856]
                                tunnel: w815 -> [w819 w825 w835 w842 w848 w852]
                                tunnel: 1.0 ("Flowrate(ul/min)") -> [w818 w824 w833 w839 w845 w851]
                                frame #0 {
                                n615 = Index Array(array=w819, index=0) -> (element=w822:dbl)
                                n616 = Greater Than 0?(x=w822) -> (x > 0?=w821:bool)
                                n617 = case shown="True" w821 {
                                tunnel: w820 -> [_ _]
                                tunnel: w818 -> [_ _]
                                frame False {
                                }
                                frame True {
                                }
                                }
                                }
                                frame #1 {
                                n618 = Index Array(array=w825, index=1) -> (element=w827:dbl)
                                n619 = Greater Than 0?(x=w827) -> (x > 0?=w826:bool)
                                n620 = case shown="True" w826 {
                                tunnel: w824 -> [_ w831]
                                tunnel: w829 -> [_ w830]
                                frame False {
                                }
                                frame True {
                                n621 = local read "Syringe_pump?"() -> (w832:bool)
                                n622 = case shown="False" w832 {
                                tunnel: w831 -> [_ _]
                                tunnel: w830 -> [_ _]
                                frame False {
                                }
                                frame True {
                                }
                                }
                                }
                                }
                                }
                                frame #2 {
                                n623 = Index Array(array=w835, index=2) -> (element=w836:dbl)
                                n624 = Greater Than 0?(x=w836) -> (x > 0?=w834:bool)
                                n625 = case shown="True" w834 {
                                tunnel: w838 -> [_ _]
                                tunnel: w833 -> [_ _]
                                frame False {
                                }
                                frame True {
                                }
                                }
                                }
                                frame #3 {
                                n626 = Index Array(array=w842, index=3) -> (element=w843:dbl)
                                n627 = Greater Than 0?(x=w843) -> (x > 0?=w841:bool)
                                n628 = case shown="True" w841 {
                                tunnel: w840 -> [_ _]
                                tunnel: w839 -> [_ _]
                                frame False {
                                }
                                frame True {
                                (unwired) "f" ("Pump Address")
                                }
                                }
                                }
                                frame #4 {
                                n629 = Index Array(array=w848, index=4) -> (element=w849:dbl)
                                n630 = Greater Than 0?(x=w849) -> (x > 0?=w847:bool)
                                n631 = case shown="True" w847 {
                                tunnel: w846 -> [_ _]
                                tunnel: w845 -> [_ _]
                                frame False {
                                }
                                frame True {
                                }
                                }
                                }
                                frame #5 {
                                n632 = Index Array(array=w852, index=5) -> (element=w854:dbl)
                                n633 = Greater Than 0?(x=w854) -> (x > 0?=w853:bool)
                                n634 = case shown="True" w853 {
                                tunnel: w856 -> [_ _]
                                tunnel: w851 -> [_ _]
                                frame False {
                                }
                                frame True {
                                }
                                }
                                }
                                }
                                }
                                frame #1 {
                                n635 = while {
                                stop <- w862 stop-if-true
                                n636 = local read "Phase_Sensor_voltage"() -> (w857:dbl)
                                n637 = script code="organic_phase = 0;\nif start_phase_time \n   start_phase_timer = tic;\n   start_phase_time = 0;\nelse\n  %ignore phase sensor values\n  %if not(phase_sensor_val >2.9 && phase_sensor_val <3.8)\n    %    start_phase_timer = tic;\n   %end\n\n   end_phase_time =  toc(start_phase_timer )\n\n   if end_phase_time > 2\n       organic_phase = 1;\n       start_phase_time = 1;\n   end\n\nend"("phase_sensor_val"=w857) -> ("organic_phase"=w859:dbl)  [unwired: 1 in, 1 out]
                                n638 = local read "Stop"() -> (w861:bool)
                                n639 = Not Equal To 0?(x=w859) -> (x != 0?=w860:bool)
                                n640 = Or(x=w860, y=w861) -> (x .or. y?=w862:bool)
                                n641 = Wait (ms)(milliseconds to wait=u32 300) -> ()  [unwired: 1 out]
                                }
                                }
                                frame #2 {
                                n642 = local read "Stop"() -> (w864:bool)
                                n643 = Not(x=w864) -> (.not. x?=w863:bool)
                                n644 = local read "Sample Valve COMM::Port"() -> (w865:refnum<visa-resource-name>)
                                n645 = case shown="True" w863 {
                                tunnel: w865 -> [_ _]
                                frame False {
                                }
                                frame True {
                                }
                                }
                                }
                                frame #3 {
                                n646 = local read "Stop"() -> (w869:bool)
                                n647 = local read "Bay Parameters"() -> (w866:T2)
                                n648 = Unbundle By Name(w866) -> ("Hplc Wait time(min)"=w867:dbl)
                                n649 = Not(x=w869) -> (.not. x?=w868:bool)
                                n650 = case shown="True" w868 {
                                tunnel: w867 -> [_ w870]
                                tunnel: w866 -> [_ _]
                                frame False {
                                (unwired) errorcluster {"status"=FALSE, "code"=0, "source"=""} ("error out")
                                }
                                frame True {
                                n651 = flat-sequence {
                                tunnel: w870 -> [w872]
                                frame #0 {
                                # "Wait till for HPLC Method"
                                n652 = script code="start = tic;"() -> ("??"=w871:errorcluster)  [unwired: 1 in]
                                n653 = while {
                                tunnel: w872 -> [w874]
                                tunnel: w871 -> [w873]
                                stop <- w880 stop-if-true
                                n654 = Multiply(x=w874, y=60.0) -> (x*y=w875:dbl)
                                n655 = script code="end1 = toc(start);\nflush_time = 0;\nif end1 > hplc_wait_time\n   flush_time = 1;\nend"("??"=w873, "hplc_wait_time"=w875) -> ("flush_time"=w877:dbl)  [unwired: 1 out]
                                n656 = local read "Stop"() -> (w879:bool)
                                n657 = Not Equal To 0?(x=w877) -> (x != 0?=w878:bool)
                                n658 = Or(x=w878, y=w879) -> (x .or. y?=w880:bool)
                                }
                                }
                                frame #1 {
                                }
                                frame #2 {
                                n659 = Wait (ms)(milliseconds to wait=u32 30000) -> ()  [unwired: 1 out]
                                }
                                frame #3 {
                                }
                                }
                                }
                                }
                                }
                                frame #4 {
                                }
                                frame #5 {
                                n660 = One Button Dialog(message="Press OK to Analyze Data", button name ("OK")="OK" ("Left Button Text (\"Yes\")")) -> ()  [unwired: 1 out]
                                n661 = disable-structure shown="Disabled" {
                                frame Disabled {
                                n662 = flat-sequence {
                                tunnel: w885 -> [w890]
                                tunnel: [w890] -> w884
                                frame #0 {
                                n663 = Wait (ms)(milliseconds to wait=u32 500) -> ()  [unwired: 1 out]
                                }
                                }
                                n664 = call-poly <vilib>:"Digital Write.vi"("Output Value"=FALSE, "DO Channel"=u8 22) -> ("LINX Resource"=w885:T13)  [unwired: 8 in, 1 out]
                                n665 = call-poly <vilib>:"Digital Write.vi"("Output Value"=TRUE, "DO Channel"=u8 22, "LINX Resource"=w884) -> ()  [unwired: 7 in, 2 out]
                                }
                                frame Enabled {
                                }
                                }
                                }
                                }
                                }
                                }
                              }
                              frame #2 {
                                n666 = local read "Stop"() -> (w893:bool)
                                n667 = local write "HPLC Analysis"(TRUE ("HPLC Analysis")) -> ()
                                n668 = Not(x=w893) -> (.not. x?=w892:bool)
                                n669 = case shown="True" w892 {
                                frame False {
                                }
                                frame True {
                                n670 = script code="C_measured =Conc;\nFvalues(end +1,:) = [Conc];"() -> ()  [unwired: 1 in, 1 out]
                                }
                                }
                              }
                            }
                          }
                          frame #4 {
                            n671 = local read "Stop"() -> (w896:bool)
                            n672 = Not(x=w896) -> (.not. x?=w895:bool)
                            n673 = case shown="True" w895 {
                              tunnel: [1.0 w907] -> w897
                              frame False {
                              }
                              frame True {
                                # "Save data to excel file"
                                n674 = local read "Bay Parameters"() -> (w905:T2)
                                n675 = Unbundle By Name(w905) -> ("Total Number of Experiments 2"=w904:dbl)
                                n676 = script code="analyze_labview_results"("ncall"=w904) -> ("terminate"=w907:dbl, "ncall0"=w906:dbl, "experiment_history"=w902:dbl[][], "Pbest"=w900:dbl[], "Tbest"=w901:dbl[], "best_exp_num"=w899:dbl)  [unwired: 1 in, 1 out]
                                n677 = local write "Flowrates(ul/min)_best"(w900) -> ()
                                n678 = local write "temperature_best"(w901) -> ()
                                n679 = local write "best_exp_num"(w899) -> ()
                                n680 = local write "Current Experiment"(w906) -> ()
                                n681 = local write "Total Number of Experiments"(w904) -> ()
                                n682 = call-poly <vilib>:"Array To Matrix.vi"("Real 2D Array"=w902) -> ("Real Matrix"=w903:T12)
                                n683 = local write "experiment history"(w903) -> ()
                              }
                            }
                          }
                          frame #5 {
                            n684 = local read "Num_exp_till_pause"() -> (w909:i32)
                            n685 = Increment(x=w909) -> (x+1=w908:i32)
                            n686 = local write "Num_exp_till_pause"(w908) -> ()
                          }
                          frame #6 {
                            # "Pause System"
                            n687 = local read "Bay Parameters"() -> (w917:T2)
                            n688 = Unbundle By Name(w917) -> ("Num_conditons_per_wait"=w916:dbl)
                            n689 = local read "Num_exp_till_pause"() -> (w915:i32)
                            n690 = Equal?(x=w916, y=w915) -> (x = y?=w914:bool)
                            n691 = local read "Run_Stop_cluster"() -> (w911:T7)
                            n692 = Unbundle By Name(w911) -> ("Stop Run Button"=w913:bool)
                            n693 = Or(x=w913, y=w914) -> (x .or. y?=w912:bool)
                            n694 = case shown="True" w912 {
                              tunnel: w916 -> [w920 _]
                              tunnel: w915 -> [w921 _]
                              tunnel: w911 -> [_ w923]
                              frame False {
                                n695 = Greater?(x=w921, y=w920) -> (0:w919:bool)
                                n696 = case shown="True" w919 {
                                frame False {
                                }
                                frame True {
                                n697 = local write "Num_exp_till_pause"(0 ("Num_exp_till_pause")) -> ()
                                }
                                }
                              }
                              frame True {
                                n698 = flat-sequence {
                                tunnel: w923 -> [w948]
                                frame #0 {
                                w927 = string[] ["e", "f", "g", "h", "i", "j"]
                                # "Turn off pumps and stop controling temperature"
                                n699 = stacked-sequence {
                                frame #0 {
                                n700 = local write "Temperature Control 1"(FALSE ("Temperature Control 1")) -> ()
                                }
                                frame #1 {
                                n701 = local write "Temperature Control 2"(FALSE ("Temperature Control 2")) -> ()
                                }
                                frame #2 {
                                n702 = local write "Temperature Control 3"(FALSE ("Temperature Control 3")) -> ()
                                }
                                frame #3 {
                                n703 = local write "Temperature Control 4"(FALSE ("Temperature Control 4")) -> ()
                                }
                                frame #4 {
                                n704 = local write "Temperature Control 5"(FALSE ("Temperature Control 5")) -> ()
                                }
                                }
                                n705 = local read "COMM Port:: Harvard Syringe Pump"() -> (w925:refnum<visa-resource-name>)
                                n706 = local read "Syringe_pump?"() -> (w924:bool)
                                n707 = local read "COMM Port :: Milligat Pumps"() -> (w926:refnum<visa-resource-name>)
                                n708 = Array Size(array=w927) -> (size(s)=w928:i32)
                                n709 = case shown="True" w924 {
                                tunnel: w925 -> [_ _]
                                frame False {
                                }
                                frame True {
                                }
                                }
                                n710 = for {
                                N: w928 -> [_]
                                tunnel: w927 -> [_] mode=indexing
                                tunnel: w926 -> [_]
                                }
                                }
                                frame #1 {
                                n711 = local read "Stop"() -> (w936:bool)
                                n712 = Not(x=w936) -> (.not. x?=w935:bool)
                                n713 = case shown="True" w935 {
                                frame False {
                                }
                                frame True {
                                n714 = while {
                                stop <- w942 stop-if-true
                                # "Wait till user confirms system resume"
                                n715 = Two Button Dialog(message="System is currently paused. Refill Syringes, flush lines, then press OK to continue optimization.\nOr Redo to repeat condition ", 1:"REDO" ("F button name (\"Cancel\")"), 2:"OK" ("Left Button Text (\"Yes\")")) -> (T button?=w938:bool)
                                n716 = case shown="False" w938 {
                                tunnel: [TRUE TRUE] -> w937
                                frame False {
                                n717 = script code="redo = true;"() -> ()  [unwired: 1 in, 1 out]
                                }
                                frame True {
                                }
                                }
                                n718 = local read "Stop"() -> (w943:bool)
                                n719 = Or(x=w937, y=w943) -> (x .or. y?=w942:bool)
                                }
                                }
                                }
                                n720 = local write "stop_xl_write"(TRUE ("stop_xl_write")) -> ()
                                }
                                frame #2 {
                                n721 = local write "Num_exp_till_pause"(0 ("Num_exp_till_pause")) -> ()
                                n722 = Bundle By Name(cluster=w948, "Stop Run Button"=FALSE) -> (w946:T7)
                                n723 = local write "Run_Stop_cluster"(w946) -> ()
                                }
                                }
                              }
                            }
                          }
                          frame #7 {
                            w951 = FALSE
                            n724 = local write "Equlibrating Temperature"(w951) -> ()
                            n725 = local write "Calculate condition"(w951) -> ()
                            n726 = local write "Flushing System"(w951) -> ()
                            n727 = local write "HPLC Analysis"(w951) -> ()
                            n728 = local write "stop_xl_write"(TRUE ("stop_xl_write")) -> ()
                          }
                        }
                        n729 = while {
                          stop <- w978 stop-if-true
                          n730 = flat-sequence {
                            frame #0 {
                              n731 = script code="save_excel_time_data;"() -> ()  [unwired: 1 in, 1 out]
                            }
                            frame #1 {
                              n732 = Wait (ms)(milliseconds to wait=u32 30000) -> ()  [unwired: 1 out]
                            }
                          }
                          n733 = local read "Stop"() -> (w979:bool)
                          n734 = local read "stop_xl_write"() -> (w977:bool)
                          n735 = Or(x=w977, y=w979) -> (x .or. y?=w978:bool)
                        }
                      }
                    }
                  }
                }
                n736 = Greater?(x=w564, y=w565) -> (0:w571:bool)
                n737 = Equal?(x=w569, y=1.0) -> (x = y?=w566:bool)
                n738 = local read "Stop"() -> (w572:bool)
                n739 = Or(x=w572, y=w571) -> (x .or. y?=w568:bool)
                n740 = Or(x=w566, y=w568) -> (x .or. y?=w567:bool)
                n741 = case shown="True" w566 {
                  frame False {
                  }
                  frame True {
                    w576 = u16 2 items=["System  Error", "System Running", "System Standby"] ("System Status")
                    n742 = local write "Stop"(TRUE ("Stop")) -> ()
                    n743 = local write "System Status"(w576) -> ()
                  }
                }
                "Optimization_loop_index" <- w573
              }
            }
          }
          n744 = while {
            stop <- w1076 stop-if-true
            n745 = local read "Temperature Control 3"() -> (w1075:bool)
            n746 = local read "running?"() -> (w1074:bool)
            n747 = And(x=w1074, y=w1075) -> (x .and. y?=w1071:bool)
            n748 = And(x=w1071, y=FALSE) -> (x .and. y?=w1072:bool)
            n749 = case shown="True" w1072 {
              frame False {
                n750 = local write "Temp SS? 3"(TRUE) -> ()
              }
              frame True {
                # "Bay 3 Temperature Controller"
                n751 = local read "Temperature SP 3"() -> (w1079:dbl)
                n752 = local read "Temperature 3"() -> (w1082:dbl)
                n753 = Subtract(x=w1082, y=w1079) -> (x-y=w1091:dbl)
                n754 = Absolute Value(x=w1091) -> (abs(x)=w1093:dbl)
                n755 = Less Or Equal?(x=w1093, y=1.2) -> (x <= y?=w1090:bool)
                n756 = local write "Temp SS? 3"(w1090) -> ()
                n757 = local read "SSR Duration 3"() -> (w1100:dbl)
                n758 = call-poly <vilib>:"PID Online Autotuning.vi"("setpoint"=w1079, "manipulated variable"=w1100, "autotuning parameters"=T9 {"type of controller"=enum."PID", "relay cycles"=3, "relay amplitude"=1.0, "control specifications"=enum."Normal", "PV noise level"=0.1} ("Autotuning Parameters R1"), "process variable"=w1082, "PID gains in"=T8 {"Proportional gain Kc"=0.38538, "Integral time Ti (sec)"=0.524375, "Derivative time Ti (sec)"=0.12585} ("PID gains 2")) -> ("setpoint out"=w1098:dbl, "process variable out"=w1099:dbl, "PID gains out"=w1102:T11)  [unwired: 6 in, 2 out]
                n759 = Greater?(x=w1079, y=w1082) -> (0:w1089:bool)
                n760 = call <vilib>:"PID Autotuning (Temperature).vi"("desired temperature"=w1098, "measured temperature"=w1099, "PID gains in"=w1102, "output range"=cluster{"output high":dbl, "output low":dbl} {"output high"=3.0, "output low"=-1.0} ("Output range")) -> ("output"=w1095:dbl)  [unwired: 12 in, 3 out]
                n761 = Multiply(x=1000.0, y=w1095) -> (x*y=w1097:dbl)
                n762 = local write "SSR Duration 3"(w1095) -> ()
                n763 = Greater Than 0?(x=w1097) -> (x > 0?=w1088:bool)
                n764 = And(x=w1088, y=w1089) -> (x .and. y?=w1086:bool)
                n765 = Subtract(x=w1082, y=10.0) -> (x-y=w1084:dbl)
                n766 = Less?(x=w1084, y=w1079) -> (x < y?=w1087:bool)
                n767 = And(x=w1087, y=w1086) -> (x .and. y?=w1085:bool)
                n768 = case shown="True" w1085 {
                  tunnel: [errorcluster {"status"=FALSE, "code"=0, "source"=""} ("error out") w1113] -> _
                  tunnel: 4 -> [_ w1111]
                  tunnel: w1097 -> [w1108 w1112]
                  tunnel: [0.0 w1115] -> w1080
                  tunnel: w1079 -> [_ w1114]
                  frame False {
                    n769 = Absolute Value(x=w1108) -> (abs(x)=w1109:dbl)
                    n770 = Wait (ms)(milliseconds to wait=w1109) -> ()  [unwired: 1 out]
                  }
                  frame True {
                    n771 = call "TurnOnRelayArduino.vi"("channel"=w1111, "duration"=w1112) -> ("error out"=w1113:errorcluster)  [unwired: 8 in, 1 out]
                    n772 = script code="tempdiff3= SP3 - T3;\nif tempdiff3 > 10\n  if slope3 < .01\n     temp_check3 = temp_check3 + 1;\n  else\n      temp_check3 =0;\n  end\nend\n\nif temp_check3 > 9\n  temp_error3 = 1\nend"("SP3"=w1114) -> ("temp_error3"=w1115:dbl)  [unwired: 1 in, 1 out]
                  }
                }
                n773 = Not Equal To 0?(x=w1080) -> (x != 0?=w1081:bool)
                n774 = case shown="True" w1081 {
                  frame False {
                  }
                  frame True {
                    n775 = local write "Error Message"("Bay 3 Temperature Heating Error") -> ()
                  }
                }
                n776 = case shown="True" w1081 {
                  tunnel: w1081 -> [_ w1106]
                  frame False {
                  }
                  frame True {
                    n777 = local write "System Error"(w1106) -> ()
                    n778 = local write "Stop"(w1106) -> ()
                  }
                }
              }
            }
            n779 = Wait (ms)(milliseconds to wait=u32 400) -> ()  [unwired: 1 out]
            n780 = local read "Stop"() -> (w1076:bool)
          }
          n781 = while {
            stop <- w1031 stop-if-true
            n782 = local read "running?"() -> (w1029:bool)
            n783 = Wait (ms)(milliseconds to wait=u32 400) -> ()  [unwired: 1 out]
            n784 = local read "Temperature Control 4"() -> (w1030:bool)
            n785 = And(x=w1029, y=w1030) -> (x .and. y?=w1026:bool)
            n786 = And(x=w1026, y=FALSE) -> (x .and. y?=w1027:bool)
            n787 = case shown="True" w1027 {
              frame False {
                n788 = local write "Temp SS? 4"(TRUE ("Temp SS? 4")) -> ()
              }
              frame True {
                # "Bay 4 Temperature Controller"
                n789 = local read "Temperature SP 4"() -> (w1036:dbl)
                n790 = local read "Temperature 4"() -> (w1039:dbl)
                n791 = Subtract(x=w1039, y=w1036) -> (x-y=w1046:dbl)
                n792 = Absolute Value(x=w1046) -> (abs(x)=w1048:dbl)
                n793 = Less Or Equal?(x=w1048, y=1.2) -> (x <= y?=w1045:bool)
                n794 = local write "Temp SS? 4"(w1045) -> ()
                n795 = local read "SSR Duration 4"() -> (w1049:dbl)
                n796 = call-poly <vilib>:"PID Online Autotuning.vi"("setpoint"=w1036, "manipulated variable"=w1049, "autotuning parameters"=T9 {"type of controller"=enum."PID", "relay cycles"=3, "relay amplitude"=1.0, "control specifications"=enum."Normal", "PV noise level"=0.1} ("Autotuning Parameters R1"), "process variable"=w1039, "PID gains in"=T8 {"Proportional gain Kc"=0.38538, "Integral time Ti (sec)"=0.524375, "Derivative time Ti (sec)"=0.12585} ("PID gains 2")) -> ("setpoint out"=w1051:dbl, "process variable out"=w1052:dbl, "PID gains out"=w1054:T11)  [unwired: 6 in, 2 out]
                n797 = call <vilib>:"PID Autotuning (Temperature).vi"("desired temperature"=w1051, "measured temperature"=w1052, "PID gains in"=w1054, "output range"=cluster{"output high":dbl, "output low":dbl} {"output high"=3.0, "output low"=-1.0} ("Output range")) -> ("output"=w1050:dbl)  [unwired: 12 in, 3 out]
                n798 = Subtract(x=w1039, y=10.0) -> (x-y=w1038:dbl)
                n799 = Less?(x=w1038, y=w1036) -> (x < y?=w1040:bool)
                n800 = Multiply(x=1000.0, y=w1050) -> (x*y=w1058:dbl)
                n801 = Greater?(x=w1036, y=w1039) -> (0:w1044:bool)
                n802 = Greater Than 0?(x=w1058) -> (x > 0?=w1043:bool)
                n803 = local write "SSR Duration 4"(w1050) -> ()
                n804 = And(x=w1043, y=w1044) -> (x .and. y?=w1042:bool)
                n805 = And(x=w1040, y=w1042) -> (x .and. y?=w1041:bool)
                n806 = case shown="True" w1041 {
                  tunnel: [errorcluster {"status"=FALSE, "code"=0, "source"=""} ("error out") w1068] -> _
                  tunnel: 5 -> [_ w1066]
                  tunnel: w1058 -> [w1063 w1067]
                  tunnel: w1036 -> [_ w1070]
                  tunnel: [0.0 w1069] -> w1035
                  frame False {
                    n807 = Absolute Value(x=w1063) -> (abs(x)=w1064:dbl)
                    n808 = Wait (ms)(milliseconds to wait=w1064) -> ()  [unwired: 1 out]
                  }
                  frame True {
                    n809 = call "TurnOnRelayArduino.vi"("channel"=w1066, "duration"=w1067) -> ("error out"=w1068:errorcluster)  [unwired: 8 in, 1 out]
                    n810 = script code="tempdiff4= SP4 - T4;\nif tempdiff4 > 10\n  if slope4 < .01\n     temp_check4 = temp_check4 + 1;\n  else\n      temp_check4 =0;\n  end\nend\n\nif temp_check4 > 9\n  temp_error4 = 1\nend"("SP4"=w1070) -> ("temp_error4"=w1069:dbl)  [unwired: 1 in, 1 out]
                  }
                }
                n811 = Not Equal To 0?(x=w1035) -> (x != 0?=w1034:bool)
                n812 = case shown="True" w1034 {
                  frame False {
                  }
                  frame True {
                    n813 = local write "Error Message"("Bay 4 Temperature Heating Error") -> ()
                  }
                }
                n814 = case shown="True" w1034 {
                  tunnel: w1034 -> [_ w1061]
                  frame False {
                  }
                  frame True {
                    n815 = local write "System Error"(w1061) -> ()
                    n816 = local write "Stop"(w1061) -> ()
                  }
                }
              }
            }
            n817 = local read "Stop"() -> (w1031:bool)
          }
          n818 = while {
            stop <- w560 stop-if-true
            n819 = script code="TempArr1=circshift(TempArr1,9);\nTempArr2=circshift(TempArr2,9);\nTempArr3=circshift(TempArr3,9);\nTempArr4=circshift(TempArr4,9);\nTempArr5=circshift(TempArr5,9);\n\nTempArr1(10)=T1;\nTempArr2(10)=T2;\nTempArr3(10)=T3;\nTempArr4(10)=T4;\nTempArr5(10)=T5;\n\n[slope1 temp] = polyfit([1,2,3,4,5,6,7,8,9,10]',TempArr1,1);\nslope1 = slope1(1);\n[slope2 temp] = polyfit([1,2,3,4,5,6,7,8,9,10]',TempArr2,1);\nslope2= slope2(1);\n[slope3 temp] = polyfit([1,2,3,4,5,6,7,8,9,10]',TempArr3,1);\nslope3 = slope3(1);\n[slope4 temp] = polyfit([1,2,3,4,5,6,7,8,9,10]',TempArr4,1);\nslope4 = slope4(1);\n[slope5 temp] = polyfit([1,2,3,4,5,6,7,8,9,10]',TempArr5,1);\nslope5 = slope5(1);"() -> ()  [unwired: 1 in, 1 out]
            n820 = Wait (ms)(milliseconds to wait=u32 600) -> ()  [unwired: 1 out]
            n821 = local read "Stop"() -> (w560:bool)
          }
          n822 = while {
            stop <- w986 stop-if-true
            n823 = local read "running?"() -> (w984:bool)
            n824 = local read "Temperature Control 5"() -> (w985:bool)
            n825 = And(x=w984, y=w985) -> (x .and. y?=w982:bool)
            n826 = And(x=w982, y=FALSE) -> (x .and. y?=w981:bool)
            n827 = case shown="True" w981 {
              frame False {
                n828 = local write "Temp SS? 5"(TRUE ("Temp SS? 5")) -> ()
              }
              frame True {
                # "Bay 5 Temperature Controller"
                n829 = local read "SSR Duration 5"() -> (w1004:dbl)
                n830 = local read "Temperature SP 5"() -> (w990:dbl)
                n831 = local read "Temperature 5"() -> (w993:dbl)
                n832 = Subtract(x=w993, y=w990) -> (x-y=w1001:dbl)
                n833 = Absolute Value(x=w1001) -> (abs(x)=w1003:dbl)
                n834 = Less Or Equal?(x=w1003, y=1.2) -> (x <= y?=w1000:bool)
                n835 = local write "Temp SS? 5"(w1000) -> ()
                n836 = call-poly <vilib>:"PID Online Autotuning.vi"("setpoint"=w990, "manipulated variable"=w1004, "autotuning parameters"=T9 {"type of controller"=enum."PID", "relay cycles"=3, "relay amplitude"=1.0, "control specifications"=enum."Normal", "PV noise level"=0.1} ("Autotuning Parameters R1"), "process variable"=w993, "PID gains in"=T8 {"Proportional gain Kc"=0.38538, "Integral time Ti (sec)"=0.524375, "Derivative time Ti (sec)"=0.12585} ("PID gains 2")) -> ("setpoint out"=w1006:dbl, "process variable out"=w1007:dbl, "PID gains out"=w1009:T11)  [unwired: 6 in, 2 out]
                n837 = call <vilib>:"PID Autotuning (Temperature).vi"("desired temperature"=w1006, "measured temperature"=w1007, "PID gains in"=w1009, "output range"=cluster{"output high":dbl, "output low":dbl} {"output high"=3.0, "output low"=-1.0} ("Output range")) -> ("output"=w1005:dbl)  [unwired: 12 in, 3 out]
                n838 = Multiply(x=1000.0, y=w1005) -> (x*y=w1013:dbl)
                n839 = Greater?(x=w990, y=w993) -> (0:w998:bool)
                n840 = Greater Than 0?(x=w1013) -> (x > 0?=w999:bool)
                n841 = local write "SSR Duration 5"(w1005) -> ()
                n842 = And(x=w999, y=w998) -> (x .and. y?=w996:bool)
                n843 = Subtract(x=w993, y=10.0) -> (x-y=w994:dbl)
                n844 = Greater?(x=w994, y=w990) -> (0:w997:bool)
                n845 = And(x=w997, y=w996) -> (x .and. y?=w995:bool)
                n846 = case shown="True" w995 {
                  tunnel: [errorcluster {"status"=FALSE, "code"=0, "source"=""} ("error out") w1023] -> _
                  tunnel: 6 -> [_ w1021]
                  tunnel: w1013 -> [w1018 w1022]
                  tunnel: [0.0 w1025] -> w991
                  tunnel: w990 -> [_ w1024]
                  frame False {
                    n847 = Absolute Value(x=w1018) -> (abs(x)=w1019:dbl)
                    n848 = Wait (ms)(milliseconds to wait=w1019) -> ()  [unwired: 1 out]
                  }
                  frame True {
                    n849 = call "TurnOnRelayArduino.vi"("channel"=w1021, "duration"=w1022) -> ("error out"=w1023:errorcluster)  [unwired: 8 in, 1 out]
                    n850 = script code="tempdiff5= SP5 - T5;\n\nif tempdiff5 > 10\n  if slope5 < .01\n     temp_check5 = temp_check5 + 1;\n  else\n      temp_check5 =0;\n  end\nend\n\nif temp_check5 >9\n  temp_error5 = 1\nend"("SP5"=w1024) -> ("temp_error5"=w1025:dbl)  [unwired: 1 in, 1 out]
                  }
                }
                n851 = Not Equal To 0?(x=w991) -> (x != 0?=w989:bool)
                n852 = case shown="True" w989 {
                  frame False {
                  }
                  frame True {
                    n853 = local write "Error Message"("Bay 5 Temperature Heating Error") -> ()
                  }
                }
                n854 = case shown="True" w989 {
                  tunnel: w989 -> [_ w1016]
                  frame False {
                  }
                  frame True {
                    n855 = local write "Stop"(w1016) -> ()
                    n856 = local write "System Error"(w1016) -> ()
                  }
                }
              }
            }
            n857 = Wait (ms)(milliseconds to wait=u32 400) -> ()  [unwired: 1 out]
            n858 = local read "Stop"() -> (w986:bool)
          }
        }
      }
      n859 = local read "IR Sensor Device"() -> (w51:T6)
      n860 = while {
        tunnel: errorcluster {"status"=FALSE, "code"=0, "source"=""} ("error out") -> [w126]
        tunnel: w51 -> [_]
        stop <- w144 stop-if-true
        (unwired) u8 5 ("Address")
        # "Bay 5 Temperature Read"
        # "Bay 4 Temperature Read"
        # "Bay 3 Temperature Read"
        # "Bay 2 Temperature Read"
        # "Bay 1 Temperature Read"
        n861 = local read "Stop"() -> (w144:bool)
        n862 = local read "Temperature SP 1"() -> (w125:dbl)
        n863 = call-poly <vilib>:"PID Control Input Filter.vi"("input"=w125) -> ("output"=w137:dbl)  [unwired: 4 in]
        n864 = case shown="False" FALSE {
          tunnel: w136 -> [w153 _]
          tunnel: [w153 w154] -> w141
          frame False {
            n865 = local write "Temperature 1"(w153) -> ()
          }
          frame True {
            n866 = local read "Temperature 1"() -> (w154:dbl)
          }
        }
        n867 = flat-sequence {
          tunnel: w137 -> [w163]
          tunnel: [w163] -> w136
          frame #0 {
            n868 = Wait (ms)(milliseconds to wait=u32 100) -> ()  [unwired: 1 out]
          }
        }
        n869 = local read "Temperature SP 2"() -> (w121:dbl)
        n870 = call-poly <vilib>:"PID Control Input Filter.vi"("input"=w121) -> ("output"=w135:dbl)  [unwired: 4 in]
        n871 = case shown="True" FALSE {
          tunnel: w134 -> [w151 _]
          tunnel: [w151 w152] -> w140
          frame False {
            n872 = local write "Temperature 2"(w151) -> ()
          }
          frame True {
            n873 = local read "Temperature 2"() -> (w152:dbl)
          }
        }
        n874 = flat-sequence {
          tunnel: w135 -> [w161]
          tunnel: [w161] -> w134
          frame #0 {
            n875 = Wait (ms)(milliseconds to wait=u32 100) -> ()  [unwired: 1 out]
          }
        }
        n876 = local read "Temperature SP 3"() -> (w119:dbl)
        n877 = case shown="False" FALSE {
          tunnel: w131 -> [w149 _]
          tunnel: [w149 w150] -> w133
          frame False {
            n878 = local write "Temperature 3"(w149) -> ()
          }
          frame True {
            n879 = local read "Temperature 3"() -> (w150:dbl)
          }
        }
        n880 = call-poly <vilib>:"PID Control Input Filter.vi"("input"=w119) -> ("output"=w132:dbl)  [unwired: 4 in]
        n881 = flat-sequence {
          tunnel: w132 -> [w159]
          tunnel: [w159] -> w131
          frame #0 {
            n882 = Wait (ms)(milliseconds to wait=u32 100) -> ()  [unwired: 1 out]
          }
        }
        n883 = local read "Temperature SP 4"() -> (w117:dbl)
        n884 = case shown="True" FALSE {
          tunnel: w129 -> [w147 _]
          tunnel: [w147 w148] -> w139
          frame False {
            n885 = local write "Temperature 4"(w147) -> ()
          }
          frame True {
            n886 = local read "Temperature 4"() -> (w148:dbl)
          }
        }
        n887 = call-poly <vilib>:"PID Control Input Filter.vi"("input"=w117) -> ("output"=w130:dbl)  [unwired: 4 in]
        n888 = flat-sequence {
          tunnel: w130 -> [w157]
          tunnel: [w157] -> w129
          frame #0 {
            n889 = Wait (ms)(milliseconds to wait=u32 100) -> ()  [unwired: 1 out]
          }
        }
        n890 = local read "Temperature SP 5"() -> (w116:dbl)
        n891 = flat-sequence {
          tunnel: w128 -> [w155]
          tunnel: [w155] -> w127
          frame #0 {
            n892 = Wait (ms)(milliseconds to wait=u32 100) -> ()  [unwired: 1 out]
          }
        }
        n893 = call-poly <vilib>:"PID Control Input Filter.vi"("input"=w116) -> ("output"=w128:dbl)  [unwired: 4 in]
        n894 = local write "error out"(w126) -> ()
        n895 = Build Array(w141, w140, w133, w139, w127) -> (w143:dbl[])
        n896 = Array To Cluster(array=w143) -> (cluster=→"Teperature Chart":T3)
        n897 = case shown="False" FALSE {
          tunnel: w127 -> [w145 _]
          tunnel: [w145 w146] -> w138
          frame False {
            n898 = local write "Temperature 5"(w145) -> ()
          }
          frame True {
            n899 = local read "Temperature 5"() -> (w146:dbl)
          }
        }
        n900 = script code="MATLAB script"("T1"=w141, "T2"=w140, "T3"=w133, "T4"=w139, "T5"=w138) -> ()  [unwired: 1 in, 1 out]
      }
      n901 = while {
        stop <- w81 stop-if-true
        n902 = local read "Pump setpoint(ul/min) 1"() -> (w84:dbl)
        n903 = local read "Pump setpoint(ul/min) 2"() -> (w80:dbl)
        n904 = local read "Pump setpoint(ul/min) 3"() -> (w79:dbl)
        n905 = local read "Pump setpoint(ul/min) 4"() -> (w78:dbl)
        n906 = local read "Pump setpoint(ul/min) 5"() -> (w77:dbl)
        n907 = local read "Pump setpoint(ul/min) 6"() -> (w76:dbl)
        n908 = Build Array(w84, w80, w79, w78, w77, w76) -> (w85:dbl[])
        n909 = Array To Cluster(array=w85) -> (cluster=→"Pump Setpoints Chart":T3)
        n910 = Wait (ms)(milliseconds to wait=u32 5000) -> ()  [unwired: 1 out]
        n911 = local read "Stop"() -> (w81:bool)
      }
      n912 = while {
        stop <- w65 stop-if-true
        n913 = local read "System Error"() -> (w64:bool)
        n914 = Wait (ms)(milliseconds to wait=u32 300) -> ()  [unwired: 1 out]
        n915 = case shown="False" w64 {
          tunnel: [w69 w70] -> w62
          frame False {
            w66 = u16 2 items=["System  Error", "System Running", "System Standby"] ("System Status")
            w67 = u16 1 items=["System  Error", "System Running", "System Standby"] ("System Status")
            n916 = local read "running?"() -> (w68:bool)
            n917 = Select(t=w67, s=w68, f=w66) -> (s? t:f=w69:u16)
          }
          frame True {
            w70 = u16 0 items=["System  Error", "System Running", "System Standby"] ("System Status")
          }
        }
        n918 = local read "Stop"() -> (w65:bool)
        n919 = local write "System Status"(w62) -> ()
      }
      n920 = while {
        stop <- w75 stop-if-true
        w71 = 0.0 ("Phase_Sensor_voltage")
        n921 = Wait (ms)(milliseconds to wait=u32 300) -> ()  [unwired: 1 out]
        n922 = Build Array(w71) -> (w72:dbl[])
        n923 = Array To Cluster(array=w72) -> (cluster=→"Phase Sensor Chart":T3)
        n924 = local read "Stop"() -> (w75:bool)
        "Phase_Sensor_voltage" <- w71
      }
      n925 = while {
        stop <- w59 stop-if-true
        n926 = script code="TempArrLED=circshift(TempArrLED,9);\nTempArrLED(10)=T1;\navgTemp = mean(TempArrLED);"() -> ("avgTemp"=w55:dbl)  [unwired: 1 in, 1 out]
        n927 = Wait (ms)(milliseconds to wait=u32 1000) -> ()  [unwired: 1 out]
        n928 = Greater?(x=w55, y=110.0) -> (0:w57:bool)
        n929 = case shown="True" w57 {
          frame False {
          }
          frame True {
            w61 = TRUE
            n930 = local write "Stop"(w61) -> ()
            n931 = local write "System Error"(w61) -> ()
            n932 = local write "Error Message"("Temperature in Bay 2 is above 110'C") -> ()
            n933 = script code="system_error = 1;"() -> ()  [unwired: 1 in, 1 out]
          }
        }
        n934 = local read "Stop"() -> (w59:bool)
      }
      n935 = while {
        stop <- w111 stop-if-true
        w86 = dbl[] [1.0, 1.0] ("array")
        w93 = 270
        w87 = 600
        w88 = 600
        (unwired) i32[] [14, 15, 14, 15]
        # "Read Pressure and Flowrate"
        n936 = local read "Stop"() -> (w111:bool)
        n937 = Index Array(array=w86, index=1) -> (element=w107:dbl)
        n938 = Index Array(array=w86, index=0) -> (element=w108:dbl)
        n939 = call-poly <vilib>:"PID Control Input Filter.vi"("input"=w107) -> ("output"=w100:dbl)  [unwired: 4 in]
        n940 = call-poly <vilib>:"PID Control Input Filter.vi"("input"=w108) -> ("output"=w99:dbl)  [unwired: 4 in]
        n941 = Multiply(x=104.96 ("y"), y=w100) -> (x*y=w101:dbl)
        n942 = Multiply(x=104.96 ("y"), y=w99) -> (x*y=w104:dbl)
        n943 = Subtract(x=w101, y=24.077) -> (x-y=w91:dbl)
        n944 = Subtract(x=w104, y=24.077) -> (x-y=w92:dbl)
        n945 = Build Array(w88, w87) -> (w96:i32[])
        n946 = Array To Cluster(array=w96) -> (cluster=→"Flowrate Chart":T4)
        n947 = Build Array(w92, w91) -> (w97:dbl[])
        n948 = local write "Flowrate Sensor 1"(w88) -> ()
        n949 = local write "Flowrate Sensor 2"(w87) -> ()
        n950 = local write "Pressure 1"(w92) -> ()
        n951 = local write "Pressure 2"(w91) -> ()
        n952 = Array To Cluster(array=w97) -> (cluster=→"Pressure Chart":T3)
        n953 = Wait (ms)(milliseconds to wait=u32 500) -> ()  [unwired: 1 out]
        n954 = script code="MATLAB script"("F1"=w88, "F2"=w87, "Pres1"=w92, "Pres2"=w91) -> ()  [unwired: 1 in, 1 out]
        n955 = Greater?(x=w91, y=w93) -> (0:w89:bool)
        n956 = Greater?(x=w92, y=w93) -> (0:w90:bool)
        n957 = case shown="False" w90 {
          frame False {
          }
          frame True {
            w115 = TRUE ("Stop")
            n958 = local write "System Error"(w115) -> ()
            n959 = local write "Stop"(w115) -> ()
            n960 = local write "Error Message"("Pressure Sensor 1 readings above 250psi") -> ()
            n961 = script code="system_error = 1;"() -> ()  [unwired: 1 in, 1 out]
          }
        }
        n962 = case shown="True" w89 {
          frame False {
          }
          frame True {
            w113 = TRUE ("Stop")
            n963 = local write "System Error"(w113) -> ()
            n964 = local write "Error Message"("Pressure Sensor 2 readings above 250psi") -> ()
            n965 = local write "Stop"(w113) -> ()
            n966 = script code="system_error = 1;"() -> ()  [unwired: 1 in, 1 out]
          }
        }
      }
    }
    frame #3 {
      # "Save and close xml and excel file"
      n967 = script code="if exist('xl_file','var') & exist('xlApp','var')\n  xlWorkbook.SaveAs(xl_file);\n  xlWorkbook.Close;\n  xlApp.Quit;\n  xlApp.delete;\nend"() -> ()  [unwired: 1 in, 1 out]
    }
    frame #4 {
      w1214 = string[] ["e", "f", "g", "h", "i", "j"]
      # "End communication to hardware"
      n968 = local read "Syringe_pump?"() -> (w1212:bool)
      n969 = local read "COMM Port:: Harvard Syringe Pump"() -> (w1213:refnum<visa-resource-name>)
      n970 = local read "COMM Port :: Milligat Pumps"() -> (w1216:refnum<visa-resource-name>)
      n971 = Array Size(array=w1214) -> (size(s)=w1215:i32)
      n972 = case shown="True" w1212 {
        tunnel: w1213 -> [_ _]
        frame False {
        }
        frame True {
        }
      }
      n973 = for {
        N: w1215 -> [_]
        tunnel: w1214 -> [_] mode=indexing
        tunnel: w1216 -> [_]
        n974 = Wait (ms)(milliseconds to wait=u32 300) -> ()  [unwired: 1 out]
      }
    }
    frame #5 {
      # "Display Error Messages if necessary"
      n975 = local read "Error Message"() -> (w1218:string)
      n976 = One Button Dialog(message=w1218) -> ()  [unwired: 1 in, 1 out]
    }
  }
